vi "AnVOR.vi"() -> ()   [LabVIEW 2013]
uses:
  <vilib>/vision/Measure.llb/Straight Edge Options.ctl
  <vilib>/vision/Measure.llb/Straight Edge Process.ctl
  <vilib>/vision/Measure.llb/Edge Options.ctl
  <vilib>/vision/Measure.llb/Edge Polarity.ctl
  <vilib>/Utility/error.llb/DialogType.ctl
  <vilib>/Analysis/baseanly.llb/Mean (DBL).vi
  <vilib>/Utility/file.llb/Read From Spreadsheet File (string).vi
  <vilib>/Utility/file.llb/Read From Spreadsheet File (DBL).vi
  <vilib>/Utility/file.llb/Write To Spreadsheet File (string).vi
  <vilib>/Utility/file.llb/Write To Spreadsheet File (DBL).vi
  <vilib>/Waveform/WDTFileIO.llb/ Write Waveforms to File (1D).vi
  <vilib>/vision/NI_Vision_Development_Module.lvlib
  <vilib>/Analysis/NI_AALBase.lvlib
panel:
  out "RawTemp":waveform(dbl)[][](array[waveform])
  out "FittingParameter":T1
  out "Vertical 2":i32
  out "Horizontal 2":i32
  in  "buf_vel_graph":dbl[][](array[numeric])
  in  "Close":bool
  in  "InitialCenter":cluster{dbl, dbl}
  in  "BlobPos_Mrk":cluster{dbl, dbl}[](array[cluster])
  in  "GlobalRect_Matches":sgl[](array[numeric])
  in  "Tab Control":T2(tab)
  in  "Image Flip":u32(ring)=3 items=["Horizontal Flip", "Vertical Flip", "Central Flip", "No Flip"]
  in  "Fit Options (Find Straight Edge 3)":T3={"Number of Lines"=1, "Type"=enum."First Edge Rake", "Min. Score"=1.0, "Max. Score"=1000.0, "Orientation"=0.0, "Angle Range"=60.0, "Angle Tolerance"=1.0, "Step Size"=1, "Min. SNR (db)"=200.0, "Min. Points (%)"=25.0, "Hough Iterations"=5} {"Min. Points (%)" min=0.0 max=100.0; "Min. SNR (db)" min=0.0; "Max. Score" min=0.0 max=1024.0; "Min. Score" min=0.0 max=1024.0 step=1.0}
  in  "Fit Options (Find Straight Edge 2)":T3={"Number of Lines"=1, "Type"=enum."First Edge Rake", "Min. Score"=1.0, "Max. Score"=1000.0, "Orientation"=0.0, "Angle Range"=60.0, "Angle Tolerance"=1.0, "Step Size"=1, "Min. SNR (db)"=200.0, "Min. Points (%)"=25.0, "Hough Iterations"=5} {"Min. Points (%)" min=0.0 max=100.0; "Min. SNR (db)" min=0.0; "Max. Score" min=0.0 max=1024.0; "Min. Score" min=0.0 max=1024.0 step=1.0}
  in  "Marker Edge 3":T7={"Search Direction"=0, "Edge Options"={"Edge Polarity"=0, "Kernel Size"=3, "Width"=1, "Minimum Edge Strength"=100.0, "Interpolation Type"=enum."Zero Order", "Data Processing Method"=enum."Average"}, "Show Search Area"=TRUE, "Show Search Lines"=FALSE, "Show Edges Found"=FALSE, "Show Result"=TRUE, "Search Area Color"=65280, "Search Lines Color"=255, "Edge Locations Color"=16776960, "Result Color"=31231, "Overlay Group Name"=""} {"Search Direction" items=["Left to Right", "Right to Left", "Top to Bottom", "Bottom to Top"]; "Edge Options"."Edge Polarity" items=["All Edges", "Rising Edges", "Falling Edges"]; "Edge Options"."Minimum Edge Strength" format="%.2f"; "Edge Options"."Width" step=2; "Edge Options"."Kernel Size" step=2}
  in  "Marker Edge 2":T7={"Search Direction"=3, "Edge Options"={"Edge Polarity"=0, "Kernel Size"=3, "Width"=1, "Minimum Edge Strength"=100.0, "Interpolation Type"=enum."Zero Order", "Data Processing Method"=enum."Average"}, "Show Search Area"=TRUE, "Show Search Lines"=FALSE, "Show Edges Found"=FALSE, "Show Result"=TRUE, "Search Area Color"=65280, "Search Lines Color"=255, "Edge Locations Color"=16776960, "Result Color"=16774656, "Overlay Group Name"=""} {"Search Direction" items=["Left to Right", "Right to Left", "Top to Bottom", "Bottom to Top"]; "Edge Options"."Edge Polarity" items=["All Edges", "Rising Edges", "Falling Edges"]; "Edge Options"."Minimum Edge Strength" format="%.2f"; "Edge Options"."Width" step=2; "Edge Options"."Kernel Size" step=2}
  out "Freq:":string
  in  "FPS:":u32
  in  "CalVar_VA":path caption="Calibration File:"
  in  "Y-axis":dbl=6.0
  in  "X-axis":dbl=6.0
  in  "Cal_Val:":u16(ring) items=["2013-07-05", "2012-08-30", "2012-08-30", "2012-03-17", "2012-03-16", "2012-03-15"]
  out "comp_XY":cluster{"mean":dbl, "mean":dbl, "Angle":sgl}(graph)
  in  "BCGTD":T8={"Brightness"=171.0, "Contrast"=89.0, "Gamma"=2.0, "Detection Sensitivity"=302.0} {"Detection Sensitivity" min=0 max=500 step=1 scale=0.0..500.0 scale format="%.2f"; "Gamma" min=0.1 max=10 step=0.01 scale=0.1..10.0 scale format="%.1f"; "Contrast" min=1 max=89 step=0.1 scale=0.0..89.0 scale format="%.2f"; "Brightness" min=0 max=255 step=1 scale=0.0..255.0 scale format="%.2f"}
  in  "btn_Pause":bool
  in  "btn_SaveResult":bool
  in  "btn_Reset":bool
  in  "btn_Start":bool
  in  "btn_Stop":bool
  in  "btn_Detect":bool
  in  "FrameNum":u32(slide) max=10490 scale=0.0..10490.0
  out "Img_Marker":T9(plugin-control)
  out "Img_Mod":T9(plugin-control)
  out "Img_Org":T9(plugin-control)
  in  "Video File":path
  out "Number of Matches (Pattern Matching 1)":bool
  in  "Fit Options (Find Straight Edge 1)":T3={"Number of Lines"=1, "Type"=enum."First Edge Rake", "Min. Score"=1.0, "Max. Score"=1000.0, "Orientation"=0.0, "Angle Range"=60.0, "Angle Tolerance"=1.0, "Step Size"=1, "Min. SNR (db)"=200.0, "Min. Points (%)"=25.0, "Hough Iterations"=5} {"Min. Points (%)" min=0.0 max=100.0; "Min. SNR (db)" min=0.0; "Max. Score" min=0.0 max=1024.0; "Min. Score" min=0.0 max=1024.0 step=1.0}
  in  "Marker Edge 1":T7={"Search Direction"=2, "Edge Options"={"Edge Polarity"=0, "Kernel Size"=3, "Width"=1, "Minimum Edge Strength"=100.0, "Interpolation Type"=enum."Zero Order", "Data Processing Method"=enum."Average"}, "Show Search Area"=TRUE, "Show Search Lines"=FALSE, "Show Edges Found"=FALSE, "Show Result"=TRUE, "Search Area Color"=65280, "Search Lines Color"=255, "Edge Locations Color"=16776960, "Result Color"=16711680, "Overlay Group Name"=""} {"Search Direction" items=["Left to Right", "Right to Left", "Top to Bottom", "Bottom to Top"]; "Edge Options"."Edge Polarity" items=["All Edges", "Rising Edges", "Falling Edges"]; "Edge Options"."Minimum Edge Strength" format="%.2f"; "Edge Options"."Width" step=2; "Edge Options"."Kernel Size" step=2}
  in  "Round Marker?":bool
  in  "btn_Undo":bool
  in  "Ring":u16(ring)=5 items=["HOR"=5, "VER"=6, "TOR"=7]
  in  "Point Removal":bool
  in  "Averaging Filter":enum32{"Hor", "Ver", "Tor"}(tab)
  in  "HorPk Width":i32(slide)=2 scale=0.0..30.0
  in  "HorL_Threshold":dbl
  in  "HorR_Threshold":dbl
  in  "VerL_Threshold":dbl
  in  "VerR_Threshold":dbl
  in  "VerPk Width":i32(slide)=2 scale=0.0..30.0
  in  "TorL_Threshold":dbl
  in  "TorR_Threshold":dbl
  in  "TorPk Width 3":i32(slide)=2 scale=0.0..30.0
  in  "Img_Only":bool
  in  "Tab Control 3":enum32{"Raw", "Hor_Vel", "Ver_Vel", "Tor_Vel"}(tab)
  out "Grp_ExtPos":waveform(dbl)[](graph)
  out "Grp_ExtVel":waveform(dbl)[](graph)
  in  "filterRank 2":i32=15 min=1
  out "Decaytime (Sec)":dbl
  out "Grp_ExtVel_Hor":waveform(dbl)[](graph)
  out "Grp_CycleAnal_Hor":waveform(dbl)[](graph)
  in  "Enum":enum16{"fromZero", "fromMaximum"}(ring)
  in  "filterRank":i32=20 min=1
  in  "Filp":bool
  out "Grp_ExtVel_Ver":waveform(dbl)[](graph)
  out "Grp_CycleAnal_Ver":waveform(dbl)[](graph)
  out "Grp_ExtVel_Tor":waveform(dbl)[](graph)
  out "Grp_CycleAnal_Tor":waveform(dbl)[](graph)
  in  "Tab Control 2":T10(tab)
  out "AMHV":dbl caption="MHV" format="%0.2f"
  out "#Cycles":dbl
  out "period":dbl caption="Freq" format="%.2g"
  out "Table":string[][](table)
  out "Table 2":string[][](table)
  in  "btn_Analyze":bool
  out "grph_RawPos":dbl[][](graph)
  in  "btn_Remove":bool
  in  "Raw Location:":path
  in  "Raw Data:":i32(listbox)
  in  "X-axis 2":dbl=6.0 caption="X:"
  in  "Y-axis 2":dbl=6.0 caption="Y:"
  in  "CalVar_GA":path caption="Calibration File:"
  in  "Cal_Val: 2":u16(ring) items=["2013-07-05", "2012-08-30", "2012-08-30", "2012-03-17", "2012-03-16", "2012-03-15"]
  in  "btn_SaveAnResult":bool
  in  "Filter Intensity":enum16{"0", "1", "2", "3", "4", "5"}(ring)
  out "Grp_Raw":waveform(dbl)[](graph)
  in  "Analyzed Data:":i32(listbox)
  in  "Final Location: 2":path
  out "x > 0?":bool
  in  "Cutoff?":bool
  in  "# of terms":i32=1
  out "Frequencies":dbl[](array[numeric]) format="%.2f"
  in  "index":i32=3 min=1 max=8
  in  "테이블 컨트롤":string[][](table)
  in  "Axis":u16(ring) items=["Horizontal", "Vertical"]
  in  "btn_addAvg":bool
  in  "Calibration Data:":i32(listbox)
  in  "Calibration Data Location":path
  out "grph_Calibration":waveform(dbl)(graph)
  in  "btn_rmvAvg":bool
  in  "btn_Calculate":bool
  in  "Horizontal":dbl
  in  "Vertical":dbl
  in  "CalVar_Cal":path caption="Calibration File:"
  out "CalList":i32(listbox)
  in  "btn_add2list":bool
  in  "btn_up":bool
  in  "btn_dn":bool
  in  "btn_del":bool
  in  "btn_save":bool
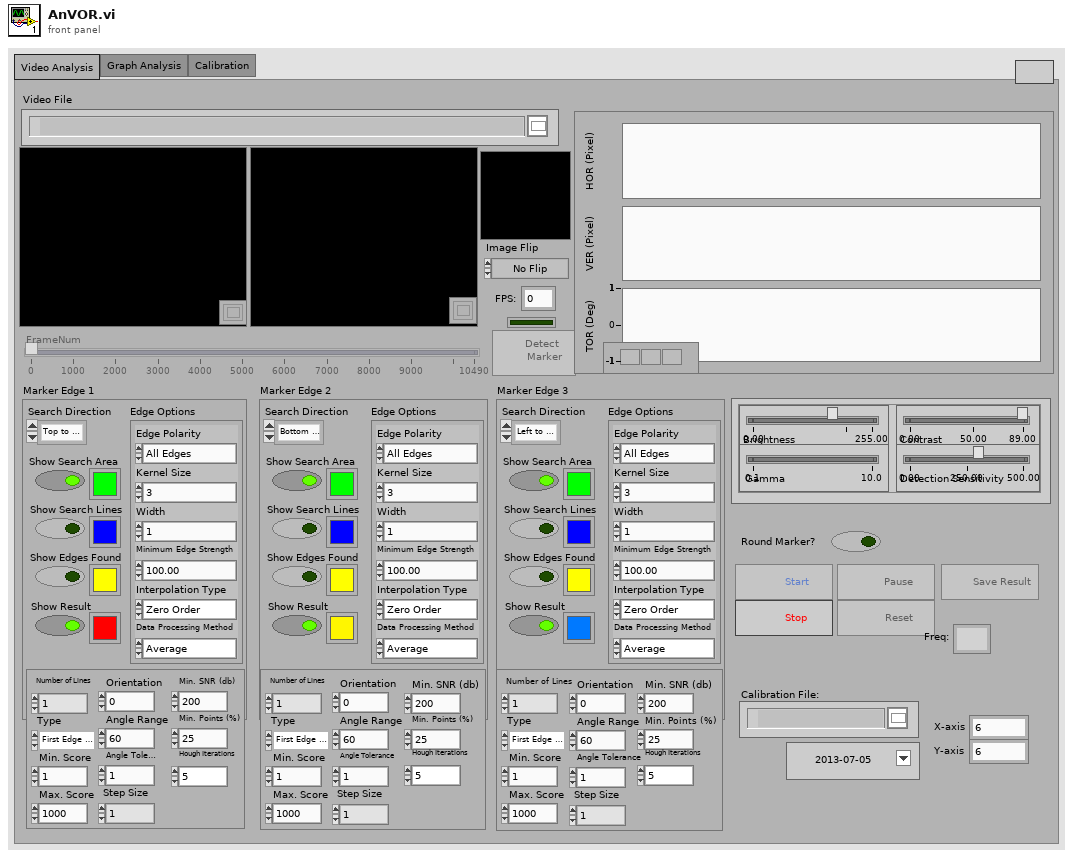
[diagram p1: front panel]
types:
  T1 = cluster{"HorL_Threshold":dbl, "HorR_Threshold":dbl, "HorPk Width":i32, "VerL_Threshold":dbl, "VerR_Threshold":dbl, "VerPk Width":i32, "TorL_Threshold 3":dbl, "TorR_Threshold":dbl, "TorPk Width 3":i32}
  T2 = enum32{"Video Analysis", "Graph Analysis", "Calibration"}
  T3 = typedef "Straight Edge Options.ctl" = cluster{"Number of Lines":i32, "Type":T4, "Min. Score":dbl, "Max. Score":dbl, "Orientation":dbl, "Angle Range":dbl, "Angle Tolerance":dbl, "Step Size":u32, "Min. SNR (db)":dbl, "Min. Points (%)":dbl, "Hough Iterations":i32}
  T4 = typedef "Straight Edge Process.ctl" = enum32{"First Edge Rake", "Best Edge Rake", "Hough Edge Rake", "First Edge Projection", "Best Edge Projection"}
  T5 = typedef "Edge Options.ctl" = cluster{"Edge Polarity":T6, "Kernel Size":u32, "Width":u32, "Minimum Edge Strength":sgl, "Interpolation Type":enum32{"Zero Order", "Bilinear", "Quadratic", "Cubic", "Bilinear Fixed"}, "Data Processing Method":enum32{"Average", "Median"}}
  T6 = typedef "Edge Polarity.ctl" = u32
  T7 = cluster{"Search Direction":u32, "Edge Options":T5, "Show Search Area":bool, "Show Search Lines":bool, "Show Edges Found":bool, "Show Result":bool, "Search Area Color":u32, "Search Lines Color":u32, "Edge Locations Color":u32, "Result Color":u32, "Overlay Group Name":string}
  T8 = cluster{"Brightness":sgl, "Contrast":sgl, "Gamma":sgl, "Detection Sensitivity":sgl}
  T9 = typedef "IMAQ Image.ctl" = refnum<image>
  T10 = enum32{"3D Analysis", "Spontaneous Nystagmus Analysis"}
  T11 = enum16{"RawDataOpen", "FinalDataOpen", "Cal2DateChange", "Calvar2Open", "RawGrpOpen", "FinalGrpOpen", "SelGrp", "RmvGrp", "SaveAnResult", "DetectMarker", "SelPlot", "Undo"}
  T12 = enum16{"Calvar3Open", "CalDataOpen", "CalGrpOpen", "AddAvg", "RmvAvg", "CalCalvar", "AddVar", "SaveVar", "Up", "Dn", "Del"}
  T13 = enum16{"VideoFileOpen", "CalvarOpen", "CalDateChange", "Adj_BCGTD", "StartTrack", "SaveResult"}
  T14 = cluster{"New Image":T9, "New Image":T9, "New Image":T9, "New Image":T9, "New Image":T9}
  T15 = typedef "LVRowAndColumnTypeDef.ctl" = cluster{"Row":i32, "Column":i32}
  T16 = typedef "DialogType.ctl" = u16
  T17 = enum16{"RawDataOpen", "FinalDataOpen", "Cal2DateChange", "Calvar2Open", "RawGrpOpen", "FinalGrpOpen", "SelGrp", "RmvGrp", "SaveAnResult", "DetectMarker", "SelPlot"}
  T18 = cluster{"Global Rectangle":i32[], "Contours":cluster{"Contour Type":u32, "ROI Type":u32, "Points":i32[]}[]}
  T19 = enum8{"Enabled", "Disabled", "Disabled and Grayed Out"}
  T20 = typedef "LVCursorListTypeDef.ctl" = cluster{"Name":string, "Color":u32, "Style":u8, "Point Style":u8, "Name Visible":bool, "Allow Drag":bool, "Cursor Mode":u32, "Plot":i32, "Index":i32, "Position":cluster{"X":dbl, "Y":dbl}, "X Scale":u32, "Y Scale":u32, "Watch Plots":i32[], "Watch All Plots":bool, "Plot Area":i32, "Label Offset":cluster{"X":dbl, "Y":dbl}}[]
  T21 = cluster{"Name":string, "Color":u32, "Style":u8, "Point Style":u8, "Name Visible":bool, "Allow Drag":bool, "Cursor Mode":u32, "Plot":i32, "Index":i32, "Position":cluster{"X":dbl, "Y":dbl}, "X Scale":u32, "Y Scale":u32, "Watch Plots":i32[], "Watch All Plots":bool, "Plot Area":i32, "Label Offset":cluster{"X":dbl, "Y":dbl}}
  T22 = cluster{"Name":string, "Color":u32, "Style":u8, "Point Style":u8, "Name Visible":bool, "Allow Drag":bool, "Cursor Mode":u32, "Plot":i32, "Index":i32, cluster{dbl, "Y":dbl}, "X Scale":u32, "Y Scale":u32, "Watch Plots":i32[], "Watch All Plots":bool, "Plot Area":i32, "Label Offset":cluster{"X":dbl, "Y":dbl}}
  T23 = cluster{"Name":string, "Color":u32, "Style":u8, "Point Style":u8, "Name Visible":bool, "Allow Drag":bool, "Cursor Mode":u32, "Plot":i32, "Index":i32, cluster{dbl, "Y":dbl}, "X Scale":u32, "Y Scale":u32, "Watch Plots":i32[], "Watch All Plots":bool, "Plot Area":i32, "Label Offset":cluster{"X":dbl, "Y":dbl}}[]
  T24 = cluster{dbl, dbl, dbl, dbl, dbl, dbl, dbl, dbl, dbl}
  T25 = enum16{"RawDataOpen", "FinalDataOpen", "Cal2DateChange", "Calvar2Open", "RawGrpOpen", "FinalGrpOpen", "SelGrp", "RmvGrp", "SaveAnResult", "DetectMarker"}
  T26 = typedef "IMAQ Rectangle" = cluster{"Left":i32, "Top":i32, "Right":i32, "Bottom":i32, "Rotation":dbl}
  T27 = typedef "AviRefnum.ctl" = refnum<k1>
  T28 = cluster{"width":u32, "height":u32, "framesPerSecond":u32, "compressionFilter":string, "hasData":bool}
  T29 = cluster{"Brightness":sgl, "Contrast":sgl, "Gamma":sgl}
  T30 = cluster{"Position":cluster{"x":sgl, "y":sgl}, "Angle":sgl, "Scale":sgl, "Score":sgl, "Bounding Box":cluster{"x":sgl, "y":sgl}[]}[]
  T31 = cluster{"Position":cluster{"x":sgl, "y":sgl}, "Angle":sgl, "Scale":sgl, "Score":sgl, "Bounding Box":cluster{"x":sgl, "y":sgl}[]}
  T32 = typedef "ROI Descriptor" = cluster{"Global Rectangle":i32[], "Contours":cluster{"ID":enum32{"External", "Internal"}, "Type":u32, "Coordinates":i32[]}[]}
  T33 = cluster{"Point1 (Pixels)":cluster{"X":sgl, "Y":sgl}, "Point2 (Pixels)":cluster{"X":sgl, "Y":sgl}, "Point1 (Real-World)":cluster{"X":sgl, "Y":sgl}, "Point2 (Real-World)":cluster{"X":sgl, "Y":sgl}, "Angle (Pixel)":dbl, "Angle (Real-World)":dbl, "Score":dbl, "Straightness":dbl, "Average SNR (db)":dbl, "Calibration Valid":bool}
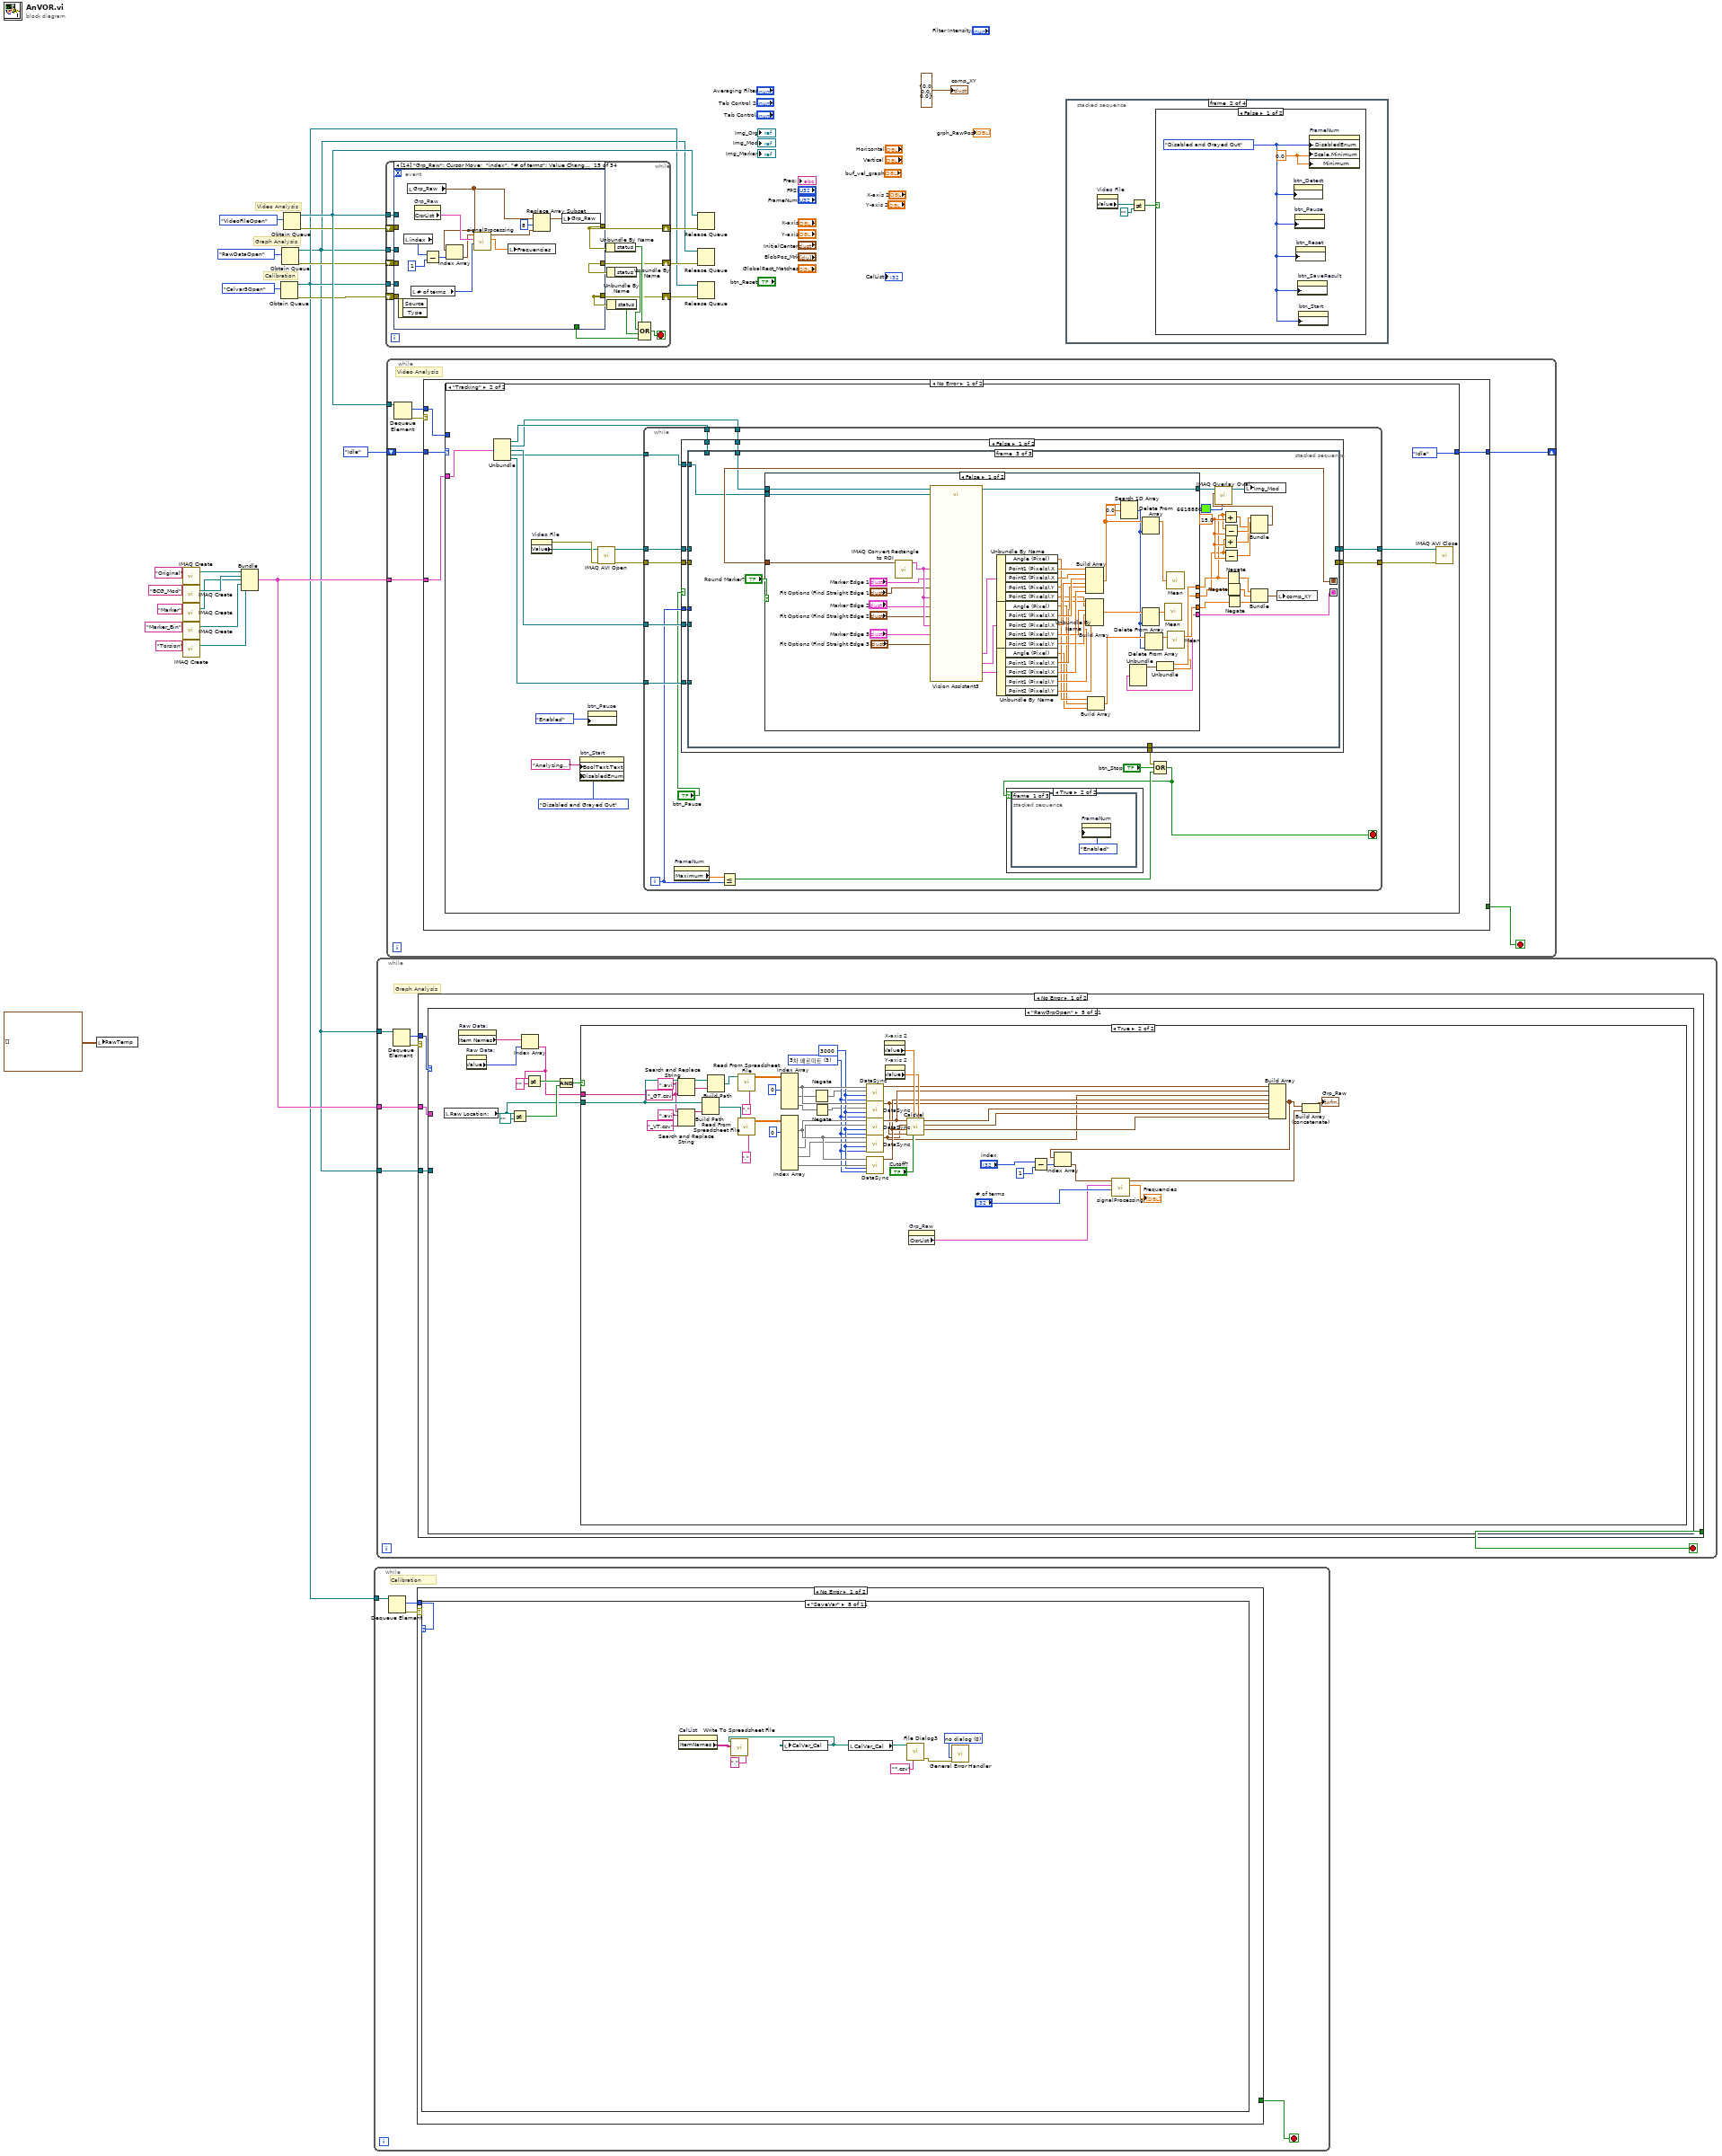
[diagram p0: block diagram]
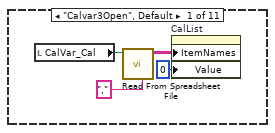
[diagram p2: hidden frame]
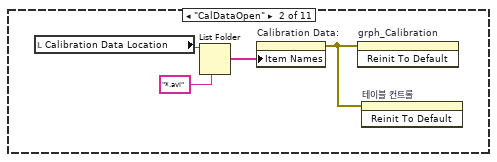
[diagram p3: hidden frame]
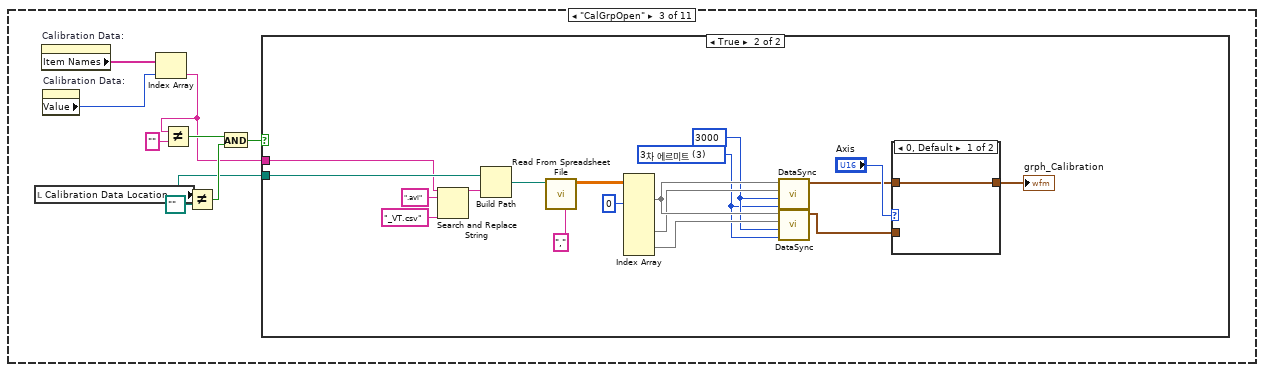
[diagram p4: hidden frame]
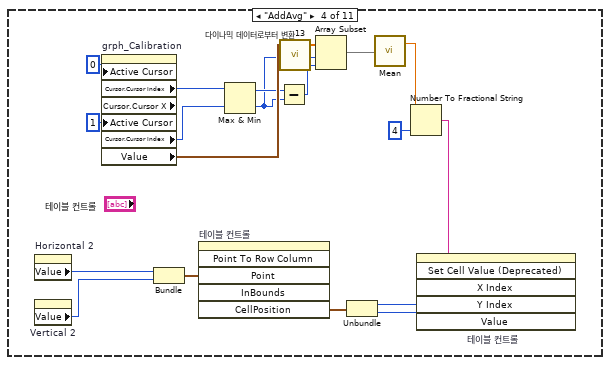
[diagram p7: hidden frame]
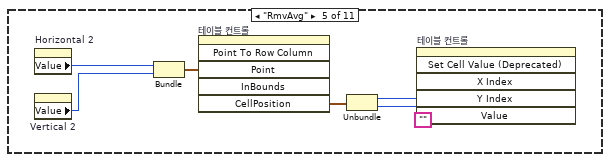
[diagram p8: hidden frame]
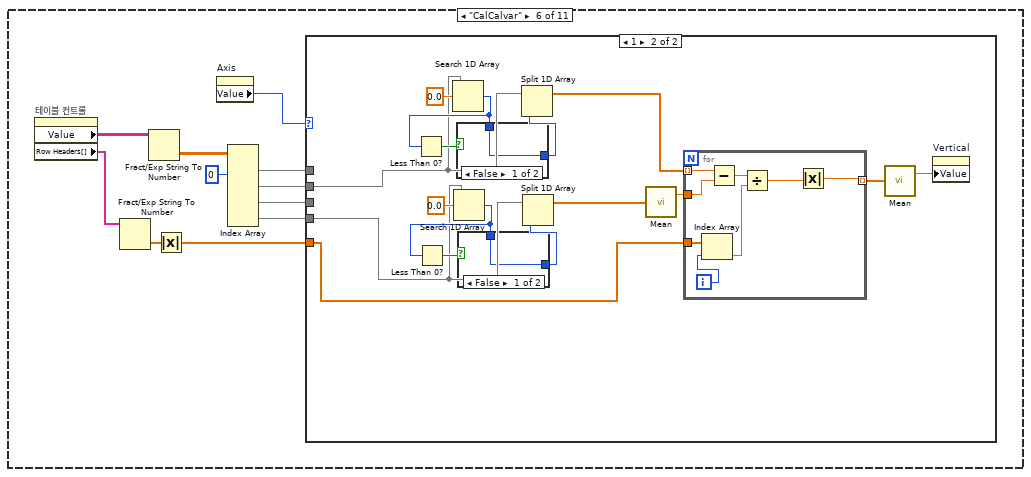
[diagram p9: hidden frame]
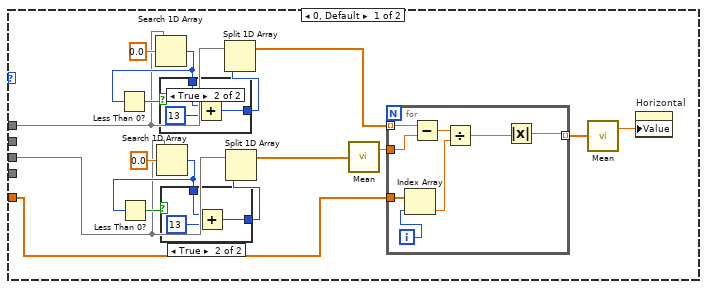
[diagram p10: hidden frame]
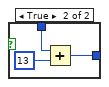
[diagram p13: hidden frame]
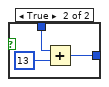
[diagram p14: hidden frame]
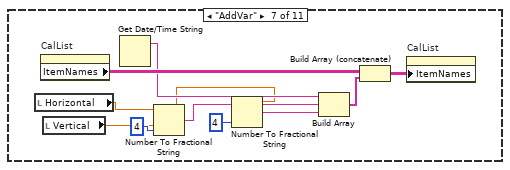
[diagram p15: hidden frame]
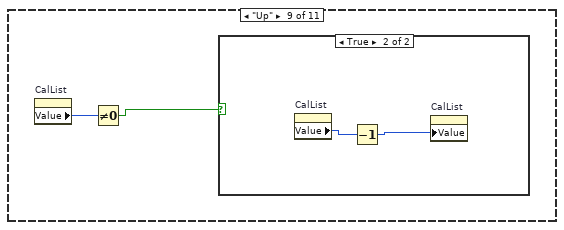
[diagram p16: hidden frame]
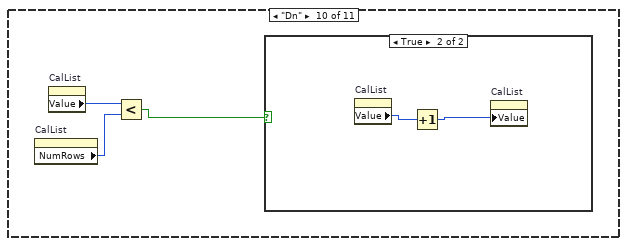
[diagram p18: hidden frame]
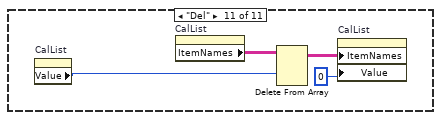
[diagram p20: hidden frame]
diagram:
  # "Calibration"
  # "Graph Analysis"
  # "Video Analysis"
  n1 = local write "RawTemp"(waveform(dbl)[][] [] ("RawTemp")) -> ()
  n2 = call "IMAQ Create"("Image Name"="Original") -> ("New Image"=w12:T9)  [unwired: 3 in, 2 out]
  n3 = call "IMAQ Create"("Image Name"="BCG_Mod") -> ("New Image"=w11:T9)  [unwired: 3 in, 2 out]
  n4 = call "IMAQ Create"("Image Name"="Marker") -> ("New Image"=w10:T9)  [unwired: 3 in, 2 out]
  n5 = call "IMAQ Create"("Image Name"="Marker_Bin") -> ("New Image"=w9:T9)  [unwired: 3 in, 2 out]
  n6 = call "IMAQ Create"("Image Name"="Torsion") -> ("New Image"=w8:T9)  [unwired: 3 in, 2 out]
  n7 = Bundle("New Image"=w12, "New Image"=w11, "New Image"=w10, "New Image"=w9, "New Image"=w8) -> (w7:T14)  [unwired: 1 in]
  n8 = Obtain Queue(element data type=T12."Calvar3Open" ("Enum")) -> (queue out=w4:refnum<queue>, error out=w16:errorcluster)  [unwired: 4 in, 1 out]
  n9 = Obtain Queue(element data type=T11."RawDataOpen" ("Enum")) -> (queue out=w3:refnum<queue>, error out=w17:errorcluster)  [unwired: 4 in, 1 out]
  n10 = Obtain Queue(element data type=T13."VideoFileOpen" ("Enum")) -> (queue out=w21:refnum<queue>, error out=w19:errorcluster)  [unwired: 4 in, 1 out]
  n11 = while {
    tunnel: w4 -> [w30]
    stop <- w27 stop-if-true
    # "Calibration"
    n12 = Dequeue Element(queue=w30) -> (element=w28:T12, error out=w29:errorcluster)  [unwired: 2 in, 2 out]
    n13 = case shown="No Error" w29 {
      tunnel: w28 -> [w31 _]
      tunnel: [_ TRUE] -> w27
      frame No Error {
        n14 = case shown="\"SaveVar\"" w31 {
          frame "Calvar3Open", Default {
            n15 = local read "CalVar_Cal"() -> (w32:path)
            n16 = call-poly <vilib>:"Read From Spreadsheet File.vi"("delimiter (\\t)"="," ("delimiter (\\t)"), "file path (dialog if empty)"=w32) -> ("all rows"=w34:string[][])  [unwired: 5 in, 4 out]
            n17 = property on="CalList" class="MCListbox (strict)"("ItemNames"=w34, "Value"=0 ("CalList")) -> ()  [unwired: 2 in, 2 out]
          }
          frame "CalDataOpen" {
            n18 = local read "Calibration Data Location"() -> (w39:path)
            n19 = List Folder(path=w39, pattern="*.avi") -> (filenames=w38:string[])  [unwired: 2 in, 3 out]
            n20 = property on="Calibration Data:" class="LstBox (strict)"("Item Names"=w38) -> (error out=w36:errorcluster)  [unwired: 2 in, 1 out]
            n21 = invoke on="grph_Calibration" class="WFGraph (엄격한)" method="Reinit To Default"(error in=w36) -> ()  [unwired: 2 in, 3 out]
            n22 = invoke on="테이블 컨트롤" class="Tbl (엄격한)" method="Reinit To Default"(error in=w36) -> ()  [unwired: 2 in, 3 out]
          }
          frame "CalGrpOpen" {
            n23 = local read "Calibration Data Location"() -> (w41:path)
            n24 = property on="Calibration Data:" class="LstBox (strict)"() -> ("Item Names"=w48:string[])  [unwired: 2 in, 2 out]
            n25 = property on="Calibration Data:" class="LstBox (strict)"() -> ("Value"=w42:i32)  [unwired: 2 in, 2 out]
            n26 = Index Array(array=w48, index=w42) -> (element=w40:string)
            n27 = Not Equal?(x=w40, y="") -> (x != y?=w45:bool)
            n28 = Not Equal?(x=w41, y=path "") -> (x != y?=w44:bool)
            n29 = And(x=w45, y=w44) -> (x .and. y?=w43:bool)
            n30 = case shown="True" w43 {
              tunnel: w41 -> [_ w66]
              tunnel: w40 -> [_ w65]
              frame False {
              }
              frame True {
                w53 = 3 items=["최근접", "선형", "스플라인", "3차 에르미트", "라그랑지"] ("method")
                w54 = 3000 ("samples")
                n31 = Search and Replace String(input string=w65, search string=".avi", replace string="_VT.csv" ("replace string (\"\")")) -> (result string=w64:string)  [unwired: 5 in, 3 out]
                n32 = Build Path(base path=w66, name or relative path=w64) -> (appended path=w60:path)
                n33 = call-poly <vilib>:"Read From Spreadsheet File.vi"("delimiter (\\t)"="," ("delimiter (\\t)"), "file path (dialog if empty)"=w60) -> ("all rows"=w59:dbl[][])  [unwired: 5 in, 4 out]
                n34 = Index Array(array=w59, index (col) #1=0 ("disabled index (col)")) -> (element #1=w57:dbl[], element #3=w56:dbl[], element #4=w55:dbl[])  [unwired: 7 in, 1 out]
                n35 = call "DataSync.vi"("method"=w53, "samples"=w54, "Y"=w56, "X"=w57) -> ("출력 웨이브폼"=w51:waveform(dbl))  [unwired: 5 in, 2 out]
                n36 = call "DataSync.vi"("method"=w53, "samples"=w54, "Y"=w55, "X"=w57) -> ("출력 웨이브폼"=w49:waveform(dbl))  [unwired: 5 in, 2 out]
                n37 = case shown="0, Default" "Axis" {
                  tunnel: [w67 w68] -> w50
                  tunnel: w51 -> [w67 _]
                  tunnel: w49 -> [_ w68]
                  frame 0, Default {
                  }
                  frame 1 {
                  }
                }
                "grph_Calibration" <- w50
              }
            }
          }
          frame "AddAvg" {
            n38 = property on="Horizontal 2" class="DigNum (strict)"() -> ("Value"=w73:i32)  [unwired: 2 in, 2 out]
            n39 = property on="Vertical 2" class="DigNum (strict)"() -> ("Value"=w72:i32)  [unwired: 2 in, 2 out]
            n40 = property on="grph_Calibration" class="WFGraph (strict)" props=["Active Cursor", "Cursor", "Cursor Index", "Cursor", "Cursor X", "Active Cursor", "Cursor", "Cursor Index", "Value"]("Active Cursor"=u32 0, "Active Cursor"=u32 1) -> ("Cursor.Cursor Index"=w83:i32, "Cursor.Cursor Index"=w85:i32, "Value"=w84:waveform(dbl))  [unwired: 2 in, 3 out]
            n41 = Bundle("Value"=w73, "Value"=w72) -> (w74:cluster{"Value":i32, "Value":i32})  [unwired: 1 in]
            n42 = invoke on="테이블 컨트롤" class="Tbl (엄격한)" method="Point To Row Column"("Point"=w74) -> ("CellPosition"=w71:T15)  [unwired: 5 in, 5 out]
            n43 = Max & Min(x=w83, y=w85) -> (max(x,y)=w82:i32, min(x,y)=w76:i32)
            n44 = Subtract(x=w82, y=w76) -> (x-y=w81:i32)
            n45 = call "다이나믹 데이터로부터 변환13"("Dynamic Data Type"=w84) -> ("Array"=w77:dbl[])  [unwired: 3 in]
            n46 = Array Subset(array=w77, index=w76, length=w81) -> (w80:dbl[])
            n47 = Unbundle(w71) -> ("Row"=w70:i32, "Column"=w69:i32)
            n48 = call-poly <vilib>:"Mean.vi"("X"=w80) -> ("mean"=w79:dbl)  [unwired: 1 out]
            n49 = Number To Fractional String(number=w79, precision (6)=i16 4) -> (F-format string=w75:string)  [unwired: 2 in]
            n50 = invoke on="테이블 컨트롤" class="Tbl (엄격한)" method="Set Cell Value (Deprecated)"("X Index"=w69, "Y Index"=w70, "Value"=w75) -> ()  [unwired: 3 in, 6 out]
          }
          frame "RmvAvg" {
            n51 = property on="Horizontal 2" class="DigNum (strict)"() -> ("Value"=w93:i32)  [unwired: 2 in, 2 out]
            n52 = property on="Vertical 2" class="DigNum (strict)"() -> ("Value"=w92:i32)  [unwired: 2 in, 2 out]
            n53 = Bundle("Value"=w93, "Value"=w92) -> (w94:cluster{"Value":i32, "Value":i32})  [unwired: 1 in]
            n54 = invoke on="테이블 컨트롤" class="Tbl (엄격한)" method="Point To Row Column"("Point"=w94) -> ("CellPosition"=w91:T15)  [unwired: 5 in, 5 out]
            n55 = Unbundle(w91) -> ("Row"=w90:i32, "Column"=w89:i32)
            n56 = invoke on="테이블 컨트롤" class="Tbl (엄격한)" method="Set Cell Value (Deprecated)"("X Index"=w89, "Y Index"=w90, "Value"="") -> ()  [unwired: 3 in, 6 out]
          }
          frame "CalCalvar" {
            n57 = property on="테이블 컨트롤" class="Tbl (strict)"() -> ("Value"=w103:string[][], "Row Headers[]"=w101:string[])  [unwired: 2 in, 2 out]
            n58 = Fract/Exp String To Number(string=w101) -> (number=w98:dbl[])  [unwired: 3 in, 1 out]
            n59 = Fract/Exp String To Number(string=w103) -> (number=w102:dbl[][])  [unwired: 3 in, 1 out]
            n60 = Absolute Value(x=w98) -> (abs(x)=w97:dbl[])
            n61 = property on="Axis" class="Ring (strict)"() -> ("Value"=w100:u16)  [unwired: 2 in, 2 out]
            n62 = Index Array(array=w102, index (col) #1=0 ("비활성화된 인덱스 (열)")) -> (element #1=w104:dbl[], element #2=w96:dbl[], element #3=w99:dbl[], element #4=w95:dbl[])  [unwired: 7 in]
            n63 = case shown="1" w100 {
              tunnel: w104 -> [w114 _]
              tunnel: w99 -> [w108 _]
              tunnel: w97 -> [w106 w140]
              tunnel: w96 -> [_ w139]
              tunnel: w95 -> [_ w138]
              frame 0, Default {
                n64 = Search 1D Array(1D array=w114, element=0.0) -> (index of element=w117:i32)  [unwired: 1 in]
                n65 = Less Than 0?(x=w117) -> (x < 0?=w116:bool)
                n66 = Search 1D Array(1D array=w108, element=0.0) -> (index of element=w110:i32)  [unwired: 1 in]
                n67 = Less Than 0?(x=w110) -> (x < 0?=w111:bool)
                n68 = case shown="True" w116 {
                  tunnel: w117 -> [w126 w129]
                  tunnel: [w126 w127] -> w118
                  frame False {
                  }
                  frame True {
                    n69 = Add(x=w129, y=13) -> (x+y=w127:i32)
                  }
                }
                n70 = case shown="True" w111 {
                  tunnel: w110 -> [w122 w125]
                  tunnel: [w122 w123] -> w109
                  frame False {
                  }
                  frame True {
                    n71 = Add(x=w125, y=13) -> (x+y=w123:i32)
                  }
                }
                n72 = Split 1D Array(array=w114, index=w118) -> (first subarray=w113:dbl[])  [unwired: 1 out]
                n73 = Split 1D Array(array=w108, index=w109) -> (first subarray=w107:dbl[])  [unwired: 1 out]
                n74 = call-poly <vilib>:"Mean.vi"("X"=w107) -> ("mean"=w121:dbl)  [unwired: 1 out]
                n75 = for {
                  tunnel: w113 -> [w137] mode=indexing
                  tunnel: w121 -> [w136]
                  tunnel: w106 -> [w134]
                  tunnel: [w130] -> w120 mode=indexing
                  i -> [w133]
                  n76 = Index Array(array=w134, index=w133) -> (element=w132:dbl)
                  n77 = Subtract(x=w137, y=w136) -> (x-y=w135:dbl)
                  n78 = Divide(x=w135, y=w132) -> (x/y=w131:dbl)
                  n79 = Absolute Value(x=w131) -> (abs(x)=w130:dbl)
                }
                n80 = call-poly <vilib>:"Mean.vi"("X"=w120) -> ("mean"=w119:dbl)  [unwired: 1 out]
                n81 = property on="Horizontal" class="DigNum (strict)"("Value"=w119) -> ()  [unwired: 2 in, 2 out]
              }
              frame 1 {
                n82 = Search 1D Array(1D array=w139, element=0.0) -> (index of element=w149:i32)  [unwired: 1 in]
                n83 = Less Than 0?(x=w149) -> (x < 0?=w148:bool)
                n84 = Search 1D Array(1D array=w138, element=0.0) -> (index of element=w143:i32)  [unwired: 1 in]
                n85 = Less Than 0?(x=w143) -> (x < 0?=w144:bool)
                n86 = case shown="False" w148 {
                  tunnel: w149 -> [w158 w161]
                  tunnel: [w158 w159] -> w150
                  frame False {
                  }
                  frame True {
                    n87 = Add(x=w161, y=13) -> (x+y=w159:i32)
                  }
                }
                n88 = case shown="False" w144 {
                  tunnel: w143 -> [w154 w157]
                  tunnel: [w154 w155] -> w142
                  frame False {
                  }
                  frame True {
                    n89 = Add(x=w157, y=13) -> (x+y=w155:i32)
                  }
                }
                n90 = Split 1D Array(array=w139, index=w150) -> (first subarray=w146:dbl[])  [unwired: 1 out]
                n91 = Split 1D Array(array=w138, index=w142) -> (first subarray=w141:dbl[])  [unwired: 1 out]
                n92 = call-poly <vilib>:"Mean.vi"("X"=w141) -> ("mean"=w153:dbl)  [unwired: 1 out]
                n93 = for {
                  tunnel: w146 -> [w169] mode=indexing
                  tunnel: w153 -> [w168]
                  tunnel: w140 -> [w166]
                  tunnel: [w163] -> w152 mode=indexing
                  i -> [w165]
                  n94 = Index Array(array=w166, index=w165) -> (element=w164:dbl)
                  n95 = Subtract(x=w169, y=w168) -> (x-y=w167:dbl)
                  n96 = Divide(x=w167, y=w164) -> (x/y=w162:dbl)
                  n97 = Absolute Value(x=w162) -> (abs(x)=w163:dbl)
                }
                n98 = call-poly <vilib>:"Mean.vi"("X"=w152) -> ("mean"=w151:dbl)  [unwired: 1 out]
                n99 = property on="Vertical" class="DigNum (strict)"("Value"=w151) -> ()  [unwired: 2 in, 2 out]
              }
            }
          }
          frame "AddVar" {
            n100 = local read "Horizontal"() -> (w177:dbl)
            n101 = property on="CalList" class="MCListbox (strict)"() -> ("ItemNames"=w179:string[][])  [unwired: 2 in, 2 out]
            n102 = local read "Vertical"() -> (w174:dbl)
            n103 = Get Date/Time String() -> (date string=w178:string)  [unwired: 3 in, 1 out]
            n104 = Number To Fractional String(number=w177, precision (6)=i16 4) -> (F-format string=w173:string)  [unwired: 2 in]
            n105 = Number To Fractional String(number=w174, precision (6)=i16 4) -> (F-format string=w172:string)  [unwired: 2 in]
            n106 = Build Array(w178, w173, w172) -> (w171:string[])
            n107 = Build Array (concatenate)(w179, w171) -> (w170:string[][])
            n108 = property on="CalList" class="MCListbox (strict)"("ItemNames"=w170) -> ()  [unwired: 2 in, 2 out]
          }
          frame "SaveVar" {
            w181 = T16 0 items=["no dialog", "OK message", "continue or stop message", "OK message + warnings", "continue/stop + warnings"] ("type of dialog (OK msg:1)")
            n109 = property on="CalList" class="MCListbox (strict)"() -> ("ItemNames"=w186:string[][])  [unwired: 2 in, 2 out]
            n110 = local read "CalVar_Cal"() -> (w184:path)
            n111 = call "File Dialog3"("start path"=w184, "pattern (all files)"="*.csv") -> ("selected path"=w180:path, "error out"=w182:errorcluster)  [unwired: 10 in, 2 out]
            n112 = call-poly <vilib>:"Write To Spreadsheet File.vi"("delimiter (\\t)"="," ("delimiter (\\t)"), "2D data"=w186, "file path (dialog if empty)"=w180) -> ()  [unwired: 5 in, 1 out]
            n113 = local write "CalVar_Cal"(w180) -> ()
            n114 = call <vilib>:"General Error Handler.vi"("type of dialog (OK msg:1)"=w181, "error in (no error)"=w182) -> ()  [unwired: 9 in, 5 out]
          }
          frame "Up" {
            n115 = property on="CalList" class="MCListbox (strict)"() -> ("Value"=w188:i32)  [unwired: 2 in, 2 out]
            n116 = Not Equal To 0?(x=w188) -> (x != 0?=w187:bool)
            n117 = case shown="True" w187 {
              frame False {
              }
              frame True {
                n118 = property on="CalList" class="MCListbox (strict)"() -> ("Value"=w190:i32)  [unwired: 2 in, 2 out]
                n119 = Decrement(x=w190) -> (x-1=w189:i32)
                n120 = property on="CalList" class="MCListbox (strict)"("Value"=w189) -> ()  [unwired: 2 in, 2 out]
              }
            }
          }
          frame "Dn" {
            n121 = property on="CalList" class="MCListbox (strict)"() -> ("NumRows"=w192:u32)  [unwired: 2 in, 2 out]
            n122 = property on="CalList" class="MCListbox (strict)"() -> ("Value"=w193:i32)  [unwired: 2 in, 2 out]
            n123 = Less?(x=w193, y=w192) -> (x < y?=w191:bool)
            n124 = case shown="True" w191 {
              frame False {
              }
              frame True {
                n125 = property on="CalList" class="MCListbox (strict)"() -> ("Value"=w195:i32)  [unwired: 2 in, 2 out]
                n126 = Increment(x=w195) -> (x+1=w194:i32)
                n127 = property on="CalList" class="MCListbox (strict)"("Value"=w194) -> ()  [unwired: 2 in, 2 out]
              }
            }
          }
          frame "Del" {
            n128 = property on="CalList" class="MCListbox (strict)"() -> ("Value"=w196:i32)  [unwired: 2 in, 2 out]
            n129 = property on="CalList" class="MCListbox (strict)"() -> ("ItemNames"=w199:string[][])  [unwired: 2 in, 2 out]
            n130 = Delete From Array(array=w199, index (row)=w196) -> (array with subset deleted=w198:string[][])  [unwired: 2 in, 1 out]
            n131 = property on="CalList" class="MCListbox (strict)"("ItemNames"=w198, "Value"=0 ("CalList")) -> ()  [unwired: 2 in, 2 out]
          }
        }
      }
      frame Error {
      }
    }
  }
  n132 = while {
    tunnel: w3 -> [w206]
    tunnel: w7 -> [w202]
    tunnel: w3 -> [w201]
    stop <- w203 stop-if-true
    # "Graph Analysis"
    n133 = Dequeue Element(queue=w206) -> (element=w204:T11, error out=w205:errorcluster)  [unwired: 2 in, 2 out]
    n134 = case shown="No Error" w205 {
      tunnel: w204 -> [w209 _]
      tunnel: [_ TRUE] -> w203
      tunnel: w202 -> [w208 _]
      tunnel: w201 -> [w207 _]
      frame No Error {
        n135 = case shown="\"RawGrpOpen\"" w209 {
          tunnel: w208 -> [_ _ _ _ _ _ w501 _ _ _ _]
          tunnel: w207 -> [_ _ w251 _ _ _ _ w535 _ _ _]
          frame "RawDataOpen", Default {
            n136 = local read "Raw Location:"() -> (w214:path)
            n137 = List Folder(path=w214, pattern="*_GT.csv") -> (filenames=w211:string[])  [unwired: 2 in, 3 out]
            n138 = for {
              tunnel: w211 -> [w216] mode=indexing
              tunnel: [w215] -> w210 mode=indexing
              n139 = Search and Replace String(input string=w216, search string="_GT.csv", replace string=".avi" ("replace string (\"\")")) -> (result string=w215:string)  [unwired: 5 in, 3 out]
            }
            n140 = property on="Raw Data:" class="LstBox (strict)"("Item Names"=w210) -> (error out=w213:errorcluster)  [unwired: 2 in, 1 out]
            n141 = invoke on="buf_vel_graph" class="Arr (strict)" method="Reinit To Default"(error in=w213) -> ()  [unwired: 2 in, 3 out]
          }
          frame "FinalDataOpen" {
            n142 = local read "Final Location: 2"() -> (w219:path)
            n143 = List Folder(path=w219, pattern="*.csv") -> (filenames=w228:string[])  [unwired: 2 in, 3 out]
            n144 = for {
              tunnel: w228 -> [w249] mode=indexing
              tunnel: [w246] -> w222 mode=indexing
              workers-P: _ -> [_]
              n145 = Search and Replace String(input string=w249, search string="_grph") -> (result string=w247:string)  [unwired: 6 in, 3 out]
              n146 = Search and Replace String(input string=w247, search string="_FitPara") -> (result string=w246:string)  [unwired: 6 in, 3 out]
            }
            n147 = Sort 1D Array(array=w222) -> (sorted array=w223:string[])
            n148 = Array Size(array=w222) -> (size(s)=w227:i32)
            n149 = for {
              N: w227 -> [_]
              shift-right: [w234] -> w225
              shift-left: w223 -> [w233]
              shift-right: [w230] -> _
              shift-left: "" -> [w238]
              shift-right: [w235] -> w226
              shift-left: 0 -> [w236]
              i -> [w232]
              stop <- w231 stop-if-true
              n150 = Index Array(array=w233, index=w232) -> (element=w230:string)
              n151 = Not Equal?(x=w230, y=w238) -> (x != y?=w237:bool)
              n152 = case shown="True" w237 {
                tunnel: w236 -> [w240 w244]
                tunnel: [w240 w245] -> w235
                tunnel: w230 -> [_ w243]
                tunnel: w233 -> [w239 w242]
                tunnel: [w239 w241] -> w234
                frame False {
                }
                frame True {
                  n153 = Replace Array Subset(array=w242, new element=w243, index=w244) -> (w241:string[])
                  n154 = Increment(x=w244) -> (x+1=w245:i32)
                }
              }
              n155 = Empty String/Path?(string/path=w230) -> (empty?=w231:bool)
            }
            n156 = Reshape Array(w225, w226) -> (w220:string[])
            n157 = property on="Analyzed Data:" class="LstBox (strict)"("Item Names"=w220) -> ()  [unwired: 2 in, 2 out]
          }
          frame "Cal2DateChange" {
            n158 = local read "CalVar_GA"() -> (w256:path)
            n159 = local read "Cal_Val: 2"() -> (w257:u16)
            n160 = property on="Grp_Raw" class="WFGraph (strict)"() -> ("Value"=w255:waveform(dbl)[])  [unwired: 2 in, 2 out]
            n161 = call "다이나믹 데이터로부터 변환3"("Dynamic Data Type"=w255) -> ("Array"=w254:dbl[])  [unwired: 3 in]
            n162 = Empty Array?(array=w254) -> (empty?=w253:bool)
            n163 = call-poly <vilib>:"Read From Spreadsheet File.vi"("delimiter (\\t)"="," ("delimiter (\\t)"), "file path (dialog if empty)"=w256) -> ("all rows"=w259:dbl[][])  [unwired: 5 in, 4 out]
            n164 = Not(x=w253) -> (.not. x?=w252:bool)
            n165 = case shown="True" w252 {
              tunnel: w251 -> [_ w268]
              frame False {
              }
              frame True {
                n166 = Enqueue Element(queue=w268, element=T17."RawGrpOpen" ("Enum")) -> (error out=w267:errorcluster)  [unwired: 2 in, 2 out]
                n167 = Enqueue Element(queue=w268, element=T17."SelGrp" ("Enum"), error in (no error)=w267) -> ()  [unwired: 1 in, 3 out]
              }
            }
            n168 = Index Array(array=w259, index (col) #1=1 ("disabled index (col)")) -> (element #1=w263:dbl[], element #2=w265:dbl[])  [unwired: 3 in]
            n169 = Reverse 1D Array(array=w263) -> (reversed array=w264:dbl[])
            n170 = Reverse 1D Array(array=w265) -> (reversed array=w266:dbl[])
            n171 = Index Array(array=w264, index=w257) -> (element=w261:dbl)
            n172 = Index Array(array=w266, index=w257) -> (element=w262:dbl)
            n173 = local write "X-axis 2"(w261) -> ()
            n174 = local write "Y-axis 2"(w262) -> ()
          }
          frame "Calvar2Open" {
            n175 = local read "CalVar_GA"() -> (w271:path)
            n176 = call-poly <vilib>:"Read From Spreadsheet File.vi"("delimiter (\\t)"="," ("delimiter (\\t)"), "file path (dialog if empty)"=w271) -> ("all rows"=w279:string[][])  [unwired: 5 in, 4 out]
            n177 = Index Array(array=w279, index (col) #1=0 ("disabled index (col)")) -> (element #1=w277:string[], element #2=w282:string[], element #3=w286:string[])  [unwired: 5 in]
            n178 = Reverse 1D Array(array=w277) -> (reversed array=w281:string[])
            n179 = Reverse 1D Array(array=w282) -> (reversed array=w283:string[])
            n180 = Reverse 1D Array(array=w286) -> (reversed array=w288:string[])
            n181 = Index Array(array=w288, index=0) -> (element=w289:string)
            n182 = Index Array(array=w281, index=0) -> (element=w274:string)
            n183 = Index Array(array=w283, index=0) -> (element=w285:string)
            n184 = property on="Cal_Val: 2" class="Ring (strict)"("Strings []"=w281) -> (error out=w276:errorcluster)  [unwired: 2 in, 1 out]
            n185 = property on="Cal_Val: 2" class="Ring (strict)"(error in=w276, "RingText.Text"=w274) -> ()  [unwired: 1 in, 2 out]
            n186 = Fract/Exp String To Number(string=w285) -> (number=w273:dbl)  [unwired: 3 in, 1 out]
            n187 = Fract/Exp String To Number(string=w289) -> (number=w272:dbl)  [unwired: 3 in, 1 out]
            n188 = local write "Y-axis 2"(w272) -> ()
            n189 = local write "X-axis 2"(w273) -> ()
          }
          frame "RawGrpOpen" {
            n190 = local read "Raw Location:"() -> (w291:path)
            n191 = property on="Raw Data:" class="LstBox (strict)"() -> ("Item Names"=w298:string[])  [unwired: 2 in, 2 out]
            n192 = property on="Raw Data:" class="LstBox (strict)"() -> ("Value"=w292:i32)  [unwired: 2 in, 2 out]
            n193 = Not Equal?(x=w291, y=path "") -> (x != y?=w294:bool)
            n194 = Index Array(array=w298, index=w292) -> (element=w290:string)
            n195 = Not Equal?(x=w290, y="") -> (x != y?=w295:bool)
            n196 = And(x=w295, y=w294) -> (x .and. y?=w293:bool)
            n197 = case shown="True" w293 {
              tunnel: w291 -> [_ w346]
              tunnel: w290 -> [_ w345]
              frame False {
              }
              frame True {
                w322 = 3 items=["최근접", "선형", "스플라인", "3차 에르미트", "라그랑지"] ("method")
                w325 = 3000 ("samples")
                n198 = Search and Replace String(input string=w345, search string=".avi", replace string="_GT.csv" ("replace string (\"\")")) -> (result string=w339:string)  [unwired: 5 in, 3 out]
                n199 = Search and Replace String(input string=w345, search string=".avi", replace string="_VT.csv" ("replace string (\"\")")) -> (result string=w344:string)  [unwired: 5 in, 3 out]
                n200 = Build Path(base path=w346, name or relative path=w344) -> (appended path=w335:path)
                n201 = Build Path(base path=w346, name or relative path=w339) -> (appended path=w337:path)
                n202 = call-poly <vilib>:"Read From Spreadsheet File.vi"("delimiter (\\t)"="," ("delimiter (\\t)"), "file path (dialog if empty)"=w335) -> ("all rows"=w333:dbl[][])  [unwired: 5 in, 4 out]
                n203 = call-poly <vilib>:"Read From Spreadsheet File.vi"("delimiter (\\t)"="," ("delimiter (\\t)"), "file path (dialog if empty)"=w337) -> ("all rows"=w334:dbl[][])  [unwired: 5 in, 4 out]
                n204 = Index Array(array=w334, index (col) #1=0 ("disabled index (col)")) -> (element #1=w330:dbl[], element #2=w320:dbl[], element #3=w319:dbl[])  [unwired: 5 in]
                n205 = Index Array(array=w333, index (col) #1=0 ("disabled index (col)")) -> (element #1=w329:dbl[], element #3=w328:dbl[], element #4=w327:dbl[], element #5=w326:dbl[])  [unwired: 9 in, 1 out]
                n206 = Negate(x=w320) -> (-x=w321:dbl[])
                n207 = Negate(x=w319) -> (-x=w318:dbl[])
                n208 = call "DataSync.vi"("method"=w322, "samples"=w325, "Y"=w321, "X"=w330) -> ("출력 웨이브폼"=w317:waveform(dbl))  [unwired: 5 in, 2 out]
                n209 = call "DataSync.vi"("method"=w322, "samples"=w325, "Y"=w318, "X"=w330) -> ("출력 웨이브폼"=w314:waveform(dbl))  [unwired: 5 in, 2 out]
                n210 = call "DataSync.vi"("method"=w322, "samples"=w325, "Y"=w328, "X"=w329) -> ("출력 웨이브폼"=w316:waveform(dbl))  [unwired: 5 in, 2 out]
                n211 = call "DataSync.vi"("method"=w322, "samples"=w325, "Y"=w327, "X"=w329) -> ("출력 웨이브폼"=w308:waveform(dbl))  [unwired: 5 in, 2 out]
                n212 = call "DataSync.vi"("method"=w322, "samples"=w325, "Y"=w326, "X"=w329) -> ("출력 웨이브폼"=w315:waveform(dbl))  [unwired: 5 in, 2 out]
                n213 = property on="X-axis 2" class="DigNum (strict)"() -> ("Value"=w324:dbl)  [unwired: 2 in, 2 out]
                n214 = property on="Y-axis 2" class="DigNum (strict)"() -> ("Value"=w323:dbl)  [unwired: 2 in, 2 out]
                n215 = call "CalcVel.vi"("CalY"=w323, "Cutoff?"="Cutoff?", "CalX"=w324, "HV"=w314, "Tor"=w315, "Ver"=w308, "Hor"=w316) -> ("TorVel"=w311:waveform(dbl), "VerVel"=w312:waveform(dbl), "HorVel"=w313:waveform(dbl))  [unwired: 2 in]
                n216 = property on="Grp_Raw" class="WFGraph (strict)"() -> ("CrsrList"=w306:T20)  [unwired: 2 in, 2 out]
                n217 = Subtract(x="index", y=1) -> (x-y=w301:i32)
                n218 = Build Array(w317, w316, w308, w315, w314, w313, w312, w311) -> (w303:waveform(dbl)[])
                n219 = Index Array(array=w303, index=w301) -> (element=w302:waveform(dbl))
                n220 = call "signalProcessing.vi"("number of terms"="# of terms", "array"=w306, "waveform in"=w302) -> ("Frequencies"=→"Frequencies":dbl[], "output waveform"=w304:waveform(dbl))  [unwired: 6 in, 1 out]
                n221 = Build Array (concatenate)(w303, w304) -> (→"Grp_Raw":waveform(dbl)[])
              }
            }
          }
          frame "SelGrp" {
            n222 = property on="Filter Intensity" class="Enum (strict)"() -> ("Value"=w470:enum16{"0", "1", "2", "3", "4", "5"})  [unwired: 2 in, 2 out]
            n223 = property on="Grp_Raw" class="WFGraph (strict)"("Active Cursor"=u32 0, "Active Cursor"=u32 1) -> ("Cursor.Cursor X"=w473:dbl, "Cursor.Cursor X"=w472:dbl, "Value"=w471:waveform(dbl)[])  [unwired: 2 in, 2 out]
            n224 = case shown="\"1\"" w470 {
              tunnel: w471 -> [w490 w492 w494 w496 w498 w500]
              tunnel: [w490 w491 w493 w495 w497 w499] -> w469
              frame "0", Default {
              }
              frame "1" {
                n225 = call "필터3"("Signal"=w492) -> ("Filtered Signal"=w491:dynamicdata)  [unwired: 9 in, 1 out]
              }
              frame "2" {
                n226 = call "필터"("Signal"=w494) -> ("Filtered Signal"=w493:dynamicdata)  [unwired: 9 in, 1 out]
              }
              frame "3" {
                n227 = call "필터2"("Signal"=w496) -> ("Filtered Signal"=w495:dynamicdata)  [unwired: 9 in, 1 out]
              }
              frame "4" {
                n228 = call "필터4"("Signal"=w498) -> ("Filtered Signal"=w497:dynamicdata)  [unwired: 9 in, 1 out]
              }
              frame "5" {
                n229 = call "필터5"("Signal"=w500) -> ("Filtered Signal"=w499:dynamicdata)  [unwired: 9 in, 1 out]
              }
            }
            n230 = Max & Min(x=w473, y=w472) -> (max(x,y)=w476:dbl, min(x,y)=w467:dbl)
            n231 = Subtract(x=w476, y=w467) -> (x-y=w468:dbl)
            n232 = Bundle By Name(cluster=T1 {"HorL_Threshold"=0.0, "HorR_Threshold"=0.0, "HorPk Width"=2, "VerL_Threshold"=0.0, "VerR_Threshold"=0.0, "VerPk Width"=2, "TorL_Threshold 3"=0.0, "TorR_Threshold"=0.0, "TorPk Width 3"=2} ("FittingPara"), "HorPk Width"="HorPk Width", "HorR_Threshold"="HorR_Threshold", "HorL_Threshold"="HorL_Threshold", "VerPk Width"="VerPk Width", "VerR_Threshold"="VerR_Threshold", "VerL_Threshold"="VerL_Threshold", "TorPk Width 3"="TorPk Width 3", "TorR_Threshold"="TorR_Threshold", "TorL_Threshold 3"="TorL_Threshold") -> (w439:T1)
            "FittingParameter" <- w439
            n233 = call "AnalyzeGraph.vi"("Grp_Raw"=w469, "start samples/time"=w467, "FittingPara"=w439, "duration"=w468) -> ("Grp_ExtVel"=w459:waveform(dbl)[], "Grp_ExtPos"=→"Grp_ExtPos":waveform(dbl)[], "Hor_CycleOut"=→"Grp_CycleAnal_Hor":waveform(dbl)[], "Table_Out"=w461:dbl[][], "Basic_Detection"=w465:cluster{"period":dbl, "mean":dbl, dbl}, "Ver_CycleOut"=→"Grp_CycleAnal_Ver":waveform(dbl)[], "SNTable_Out"=w450:dbl[][], "Tor_CycleOut"=→"Grp_CycleAnal_Tor":waveform(dbl)[])  [unwired: 2 in, 2 out]
            "Grp_ExtVel" <- w459
            n234 = Unbundle(w465) -> ("period"=→"period":dbl, "mean"=→"AMHV":dbl, →"#Cycles":dbl)
            n235 = Number To Fractional String(number=w461) -> (F-format string=→"Table":string[][])  [unwired: 3 in]
            n236 = Number To Fractional String(number=w450) -> (F-format string=→"Table 2":string[][])  [unwired: 3 in]
            n237 = Index Array(array=w459) -> (element #1=w438:waveform(dbl), element #2=w436:waveform(dbl), element #3=w458:waveform(dbl), element #4=w456:waveform(dbl))  [unwired: 4 in]
            n238 = Build Array(w438, w458) -> (→"Grp_ExtVel_Ver":waveform(dbl)[])
            n239 = Build Array(w438, w456) -> (→"Grp_ExtVel_Tor":waveform(dbl)[])
            n240 = Unbundle By Name(w436) -> ("t0"=w419:timestamp, "dt"=w372:dbl, "Y"=w367:dbl[])
            n241 = Negate(x=w367) -> (-x=w368:dbl[])
            n242 = Select(t=w368, s="Filp", f=w367) -> (s? t:f=w353:dbl[])
            n243 = Index Array(array=w353) -> (element=w418:dbl)  [unwired: 1 in]
            n244 = Array Max & Min(array=w353) -> (max value=w354:dbl)  [unwired: 3 out]
            n245 = for {
              shift-right: [w477] -> _
              shift-left: w418 -> [w479]
              tunnel: w353 -> [w478] mode=indexing
              tunnel: [w477] -> w351 mode=indexing
              n246 = Greater Than 0?(x=w478) -> (x > 0?=w480:bool)
              n247 = Select(t=w479, s=w480, f=w478) -> (s? t:f=w477:dbl)
            }
            n248 = Equal To 0?(x="Enum") -> (x = 0?=w420:bool)
            n249 = Select(t=0.0, s=w420, f=w354) -> (s? t:f=w365:dbl)
            n250 = call "Median.vi"("Rank"="filterRank", "Array in"=w351) -> ("Array out"=w349:dbl[])  [unwired: 9 in]
            n251 = Subtract(x=1.0, y=0.36787944117144233) -> (x-y=w430:dbl)
            n252 = Multiply(x=1.0, y=w349) -> (x*y=w348:dbl[])
            n253 = Negate(x=w365) -> (-x=w366:dbl)
            n254 = Select(t=w366, s="Filp", f=w365) -> (s? t:f=w364:dbl)
            n255 = call "MovingAverage.vi"("Rank"="filterRank 2", "Array in"=w348) -> ("Array out"=w352:dbl[])  [unwired: 9 in]
            n256 = Array Max & Min(array=w352) -> (min value=w361:dbl, min index (indices)=w373:i32)  [unwired: 2 out]
            n257 = Subtract(x=w365, y=w361) -> (x-y=w431:dbl)
            n258 = Multiply(x=w431, y=w430) -> (x*y=w427:dbl)
            n259 = Add(x=w361, y=w427) -> (x+y=w358:dbl)
            n260 = Negate(x=w361) -> (-x=w363:dbl)
            n261 = Negate(x=w358) -> (-x=w360:dbl)
            n262 = Select(t=w363, s="Filp", f=w361) -> (s? t:f=w362:dbl)
            n263 = for {
              tunnel: w352 -> [w486] mode=indexing
              shift-right: [w482] -> w423
              shift-left: 0 -> [w481]
              tunnel: w358 -> [w485]
              i -> [w483]
              n264 = Greater?(x=w485, y=w486) -> (0:w484:bool)
              n265 = Select(t=w483, s=w484, f=w481) -> (s? t:f=w482:i32)
            }
            n266 = Select(t=w360, s="Filp", f=w358) -> (s? t:f=w359:dbl)
            n267 = property on="Grp_ExtVel_Hor" class="WFGraph (strict)"() -> ("CrsrList"=w415:T20)  [unwired: 2 in, 2 out]
            n268 = for {
              tunnel: w353 -> [_] mode=indexing
              tunnel: w364 -> [w489]
              tunnel: w362 -> [w488]
              tunnel: [w489] -> w434 mode=indexing
              tunnel: [w488] -> w433 mode=indexing
              tunnel: [w487] -> w425 mode=indexing
              tunnel: w359 -> [w487]
            }
            n269 = Negate(x=w352) -> (-x=w357:dbl[])
            n270 = Select(t=w357, s="Filp", f=w352) -> (s? t:f=w356:dbl[])
            n271 = Multiply(x=w372, y=w423) -> (x*y=w371:dbl)
            n272 = Bundle By Name("t0"=w419, "dt"=w372, "Y"=w356) -> (w417:waveform(dbl))  [unwired: 1 in]
            n273 = Bundle By Name("t0"=w419, "dt"=w372, "Y"=w434) -> (w435:waveform(dbl))  [unwired: 1 in]
            n274 = Bundle By Name("t0"=w419, "dt"=w372, "Y"=w433) -> (w432:waveform(dbl))  [unwired: 1 in]
            n275 = Bundle By Name("t0"=w419, "dt"=w372, "Y"=w425) -> (w426:waveform(dbl))  [unwired: 1 in]
            n276 = Multiply(x=w372, y=w373) -> (x*y=w370:dbl)
            n277 = Index Array(array=w415) -> (element #1=w414:T21, element #2=w375:T21)  [unwired: 2 in]
            n278 = Subtract(x=w371, y=w370) -> (x-y=→"Decaytime (Sec)":dbl)
            n279 = Unbundle(w414) -> ("Name"=w410:string, "Color"=w409:u32, "Style"=w408:u8, "Point Style"=w407:u8, "Name Visible"=w406:bool, "Allow Drag"=w405:bool, "Cursor Mode"=w404:u32, "Plot"=w403:i32, "Index"=w400:i32, "Position"=w412:cluster{"X":dbl, "Y":dbl}, "X Scale"=w401:u32, "Y Scale"=w399:u32, "Watch Plots"=w398:i32[], "Watch All Plots"=w397:bool, "Plot Area"=w396:i32, "Label Offset"=w395:cluster{"X":dbl, "Y":dbl})
            n280 = Unbundle(w375) -> ("Name"=w378:string, "Color"=w379:u32, "Style"=w380:u8, "Point Style"=w381:u8, "Name Visible"=w382:bool, "Allow Drag"=w383:bool, "Cursor Mode"=w384:u32, "Plot"=w385:i32, "Index"=w388:i32, "Position"=w376:cluster{"X":dbl, "Y":dbl}, "X Scale"=w387:u32, "Y Scale"=w389:u32, "Watch Plots"=w390:i32[], "Watch All Plots"=w391:bool, "Plot Area"=w392:i32, "Label Offset"=w393:cluster{"X":dbl, "Y":dbl})
            n281 = Build Array(w417, w438, w436, w435, w432, w426) -> (→"Grp_ExtVel_Hor":waveform(dbl)[])
            n282 = Unbundle By Name(w412) -> ("Y"=w411:dbl)
            n283 = Unbundle By Name(w376) -> ("Y"=w377:dbl)
            n284 = Bundle(w371, "Y"=w411) -> (w402:cluster{dbl, "Y":dbl})  [unwired: 1 in]
            n285 = Bundle(w370, "Y"=w377) -> (w386:cluster{dbl, "Y":dbl})  [unwired: 1 in]
            n286 = Bundle("Name"=w410, "Color"=w409, "Style"=w408, "Point Style"=w407, "Name Visible"=w406, "Allow Drag"=w405, "Cursor Mode"=w404, "Plot"=w403, "Index"=w400, w402, "X Scale"=w401, "Y Scale"=w399, "Watch Plots"=w398, "Watch All Plots"=w397, "Plot Area"=w396, "Label Offset"=w395) -> (w394:T22)  [unwired: 1 in]
            n287 = Bundle("Name"=w378, "Color"=w379, "Style"=w380, "Point Style"=w381, "Name Visible"=w382, "Allow Drag"=w383, "Cursor Mode"=w384, "Plot"=w385, "Index"=w388, w386, "X Scale"=w387, "Y Scale"=w389, "Watch Plots"=w390, "Watch All Plots"=w391, "Plot Area"=w392, "Label Offset"=w393) -> (w374:T22)  [unwired: 1 in]
            n288 = Build Array(w394, w374) -> (w413:T23)
            n289 = property on="Grp_ExtVel_Hor" class="WFGraph (strict)"("CrsrList"=w413) -> ()  [unwired: 2 in, 2 out]
          }
          frame "DetectMarker" {
            n290 = flat-sequence {
              tunnel: w501 -> [w521]
              frame #0 {
                w515 = 15.0 ("y")
                w527 = u16 0 items=["All", "Shift Information", "Rotation Information"] ("Learn Mode")
                n291 = property on="Img_Org" class="ImageControl"() -> ("ROI"=w519:T18)  [unwired: 2 in, 2 out]
                n292 = local read "BCGTD"() -> (w520:T8)
                n293 = Unbundle(w521) -> ("New Image"=w517:T9, "New Image"=w522:T9)  [unwired: 3 out]
                n294 = Unbundle(w520) -> ("Brightness"=w525:sgl, "Contrast"=w524:sgl, "Gamma"=w523:sgl, "Detection Sensitivity"=w516:sgl)
                n295 = Bundle("Brightness"=w525, "Contrast"=w524, "Gamma"=w523) -> ()  [unwired: 1 in, 1 out]
                n296 = Unbundle(w519) -> ("Global Rectangle"=w530:i32[])  [unwired: 1 out]
                n297 = call "IMAQ Extract"("Optional Rectangle"=w530, "Image Dst"=w522, "Image Src"=w517) -> ("error out"=w529:errorcluster, "Image Dst Out"=w526:T9)  [unwired: 3 in, 4 out]
                n298 = call "IMAQ Setup Learn Pattern 2"("Learn Mode"=w527) -> ("Learn Pattern Setup Data"=w528:string)  [unwired: 1 in, 9 out]
                n299 = call "IMAQ Learn Pattern 2"("error in (no error)"=w529, "Learn Pattern Setup Data"=w528, "Image"=w526) -> ("Template Image Out"=w518:T9)  [unwired: 1 in, 7 out]
                n300 = call "Dt_Marker.vi"("ROI Descriptor"=w519, "Minimum Match Score"=w516, "Img_Mrk"=w518, "Img_Mod"=w517) -> ("Position"=w506:cluster{"x":sgl, "y":sgl}, "Img_Mod_Out"=w507:T9, "x = 0?"=w503:bool)  [unwired: 3 in, 2 out]
                n301 = Unbundle(w506) -> ("x"=w505:sgl, "y"=w504:sgl)
                n302 = Not(x=w503) -> (.not. x?=w502:bool)
                n303 = property on="Marker Detection" class="Bool (strict)"("Value"=w502) -> ()  [unwired: 2 in, 2 out]
                n304 = Add(x=w505, y=w515) -> (x+y=w512:dbl)
                n305 = Add(x=w504, y=w515) -> (x+y=w511:dbl)
                n306 = Subtract(x=w505, y=w515) -> (x-y=w514:dbl)
                n307 = Subtract(x=w504, y=w515) -> (x-y=w513:dbl)
                n308 = Bundle(w514, w513, w512, w511) -> (w510:cluster{dbl, dbl, dbl, dbl})  [unwired: 1 in]
                n309 = call "IMAQ Overlay Oval"("Color"=u32 6618880, "Bounding Rectangle"=w510, "Image"=w507) -> ("Image Out"=w509:T9)  [unwired: 7 in, 1 out]
                n310 = local write "Img_Mod"(w509) -> ()
                n311 = local write "Img_Marker"(w518) -> ()
              }
              frame #1 {
                n312 = local read "FrameNum"() -> (w532:u32)
                n313 = property on="Img_Org" class="ImageControl"("ROI"=T18 {"Global Rectangle"=[], "Contours"=[]}) -> ()  [unwired: 2 in, 2 out]
                n314 = Equal To 0?(x=w532) -> (x = 0?=w531:bool)
                n315 = case shown="True" w531 {
                  frame False {
                  }
                  frame True {
                    n316 = property on="btn_Start" class="Bool"("DisabledEnum"=T19."Enabled" ("비활성화")) -> ()  [unwired: 2 in, 2 out]
                  }
                }
              }
            }
          }
          frame "FinalGrpOpen" {
            n317 = local read "Final Location: 2"() -> (w536:path)
            n318 = property on="Analyzed Data:" class="LstBox (strict)"() -> ("Item Names"=w544:string[])  [unwired: 2 in, 2 out]
            n319 = property on="Analyzed Data:" class="LstBox (strict)"() -> ("Value"=w539:i32)  [unwired: 2 in, 2 out]
            n320 = Not Equal?(x=w536, y=path "") -> (x != y?=w540:bool)
            n321 = Index Array(array=w544, index=w539) -> (element=w537:string)
            n322 = Not Equal?(x=w537, y="") -> (x != y?=w541:bool)
            n323 = And(x=w541, y=w540) -> (x .and. y?=w538:bool)
            n324 = case shown="True" w538 {
              tunnel: w537 -> [_ w548]
              tunnel: w536 -> [_ w547]
              tunnel: w535 -> [_ w568]
              frame False {
              }
              frame True {
                w565 = u32 0 ("Active Cursor")
                n325 = Search and Replace String(input string=w548, search string=".csv" ("검색 문자열"), replace string="_grph.csv" ("대체 문자열(\"\")")) -> (result string=w572:string)  [unwired: 5 in, 3 out]
                n326 = Search and Replace String(input string=w548, search string=".csv" ("검색 문자열"), replace string="_FitPara.csv" ("대체 문자열(\"\")")) -> (result string=w549:string)  [unwired: 5 in, 3 out]
                n327 = Build Path(base path=w547, name or relative path=w549) -> (appended path=w546:path)
                n328 = Build Path(base path=w547, name or relative path=w572) -> (appended path=w571:path)
                n329 = call-poly <vilib>:"Read From Spreadsheet File.vi"("delimiter (\\t)"="," ("delimiter (\\t)"), "file path (dialog if empty)"=w546) -> ("first row"=w561:dbl[])  [unwired: 5 in, 4 out]
                n330 = call <vilib>:"Read Waveform from File.vi"("file path (dialog if empty)"=w571) -> ("all waveforms in record"=w564:waveform(dbl)[])  [unwired: 5 in, 3 out]
                n331 = property on="Grp_Raw" class="WFGraph (strict)"("Value"=w564) -> (error out=w563:errorcluster)  [unwired: 2 in, 1 out]
                n332 = Index Array(array=w561) -> (element #1=w560:dbl, element #2=w559:dbl, element #3=w558:dbl, element #4=w557:dbl, element #5=w556:dbl, element #6=w555:dbl, element #7=w554:dbl, element #8=w553:dbl, element #9=w552:dbl)  [unwired: 9 in]
                n333 = Bundle(w560, w559, w558, w557, w556, w555, w554, w553, w552) -> (w545:T24)  [unwired: 1 in]
                n334 = property on="Grp_Raw" class="WFGraph (strict)"(error in=w563, "Active Cursor"=w565, "Cursor.Cursor Index"=w565, "Active Cursor"=u32 1) -> (error out=w566:errorcluster)  [unwired: 1 in, 1 out]
                n335 = Build Path(base path=w547, name or relative path=w548) -> (appended path=w570:path)
                n336 = property on="FittingParameter" class="Clust (strict)"("Value"=w545) -> ()  [unwired: 2 in, 2 out]
                n337 = Enqueue Element(queue=w568, element=T17."SelPlot" ("Enum"), error in (no error)=w566) -> ()  [unwired: 1 in, 3 out]
                n338 = disable-structure shown="Disabled" {
                  disable-tunnel: w570 -> [w587 _]
                  frame Disabled {
                    w581 = 0 ("인덱스 (행)")
                    n339 = call-poly <vilib>:"Read From Spreadsheet File.vi"("delimiter (\\t)"="," ("delimiter (\\t)"), "format (%.3f)"="%.6f", "file path (dialog if empty)"=w587) -> ("all rows"=w578:dbl[][])  [unwired: 4 in, 4 out]
                    n340 = Index Array(array=w578, index (row) #1=w581, index (col) #1=2 ("인덱스 (행)"), index (row) #2=w581, index (col) #2=w581, index (row) #3=w581, index (col) #3=1 ("인덱스 (행)")) -> (element #1=w579:dbl, element #2=w584:dbl, element #3=w583:dbl)
                    n341 = Delete From Array(array=w578, index (row)=0 ("인덱스 (행)")) -> (array with subset deleted=w576:dbl[][])  [unwired: 2 in, 1 out]
                    n342 = property on="#Cycles" class="DigNum (strict)"("Value"=w579) -> ()  [unwired: 2 in, 2 out]
                    n343 = Number To Fractional String(number=w576) -> (F-format string=w575:string[][])  [unwired: 3 in]
                    n344 = property on="period" class="DigNum (strict)"("Value"=w584) -> ()  [unwired: 2 in, 2 out]
                    n345 = property on="AMHV" class="DigNum (strict)"("Value"=w583) -> ()  [unwired: 2 in, 2 out]
                    n346 = property on="Table" class="Tbl (strict)"("Value"=w575) -> ()  [unwired: 2 in, 2 out]
                  }
                  frame Enabled {
                  }
                }
              }
            }
          }
          frame "RmvGrp" {
            n347 = local read "RawTemp"() -> (w588:waveform(dbl)[][])
            n348 = property on="Grp_Raw" class="WFGraph (strict)"("Active Cursor"=u32 0, "Active Cursor"=u32 1, "Active Cursor"=u32 2) -> ("Cursor.Cursor Index"=w599:i32, "Cursor.Cursor Index"=w598:i32, "Value"=w590:waveform(dbl)[], "Cursor.Cursor Index"=w591:i32)  [unwired: 2 in, 2 out]
            n349 = Max & Min(x=w599, y=w598) -> (max(x,y)=w597:i32, min(x,y)=w596:i32)
            n350 = Build Array (concatenate)(w588, w590) -> (→"RawTemp":waveform(dbl)[][])
            n351 = Subtract(x=w597, y=w596) -> (x-y=w595:i32)
            n352 = case shown="True" "Point Removal" {
              tunnel: w590 -> [w619 w643]
              tunnel: w596 -> [w612 _]
              tunnel: w595 -> [w611 _]
              tunnel: [w602 w650] -> w594
              tunnel: w591 -> [_ w642]
              frame False {
                n353 = call "다이나믹 데이터로부터 변환11"("Dynamic Data Type"=w619) -> ("Waveform"=w614:waveform(dbl))  [unwired: 3 in]
                n354 = call "다이나믹 데이터로부터 변환12"("Dynamic Data Type"=w619) -> ("Waveform"=w613:waveform(dbl))  [unwired: 3 in]
                n355 = call "다이나믹 데이터로부터 변환9"("Dynamic Data Type"=w619) -> ("Waveform"=w616:waveform(dbl))  [unwired: 3 in]
                n356 = call "다이나믹 데이터로부터 변환10"("Dynamic Data Type"=w619) -> ("Waveform"=w615:waveform(dbl))  [unwired: 3 in]
                n357 = call "다이나믹 데이터로부터 변환5"("Dynamic Data Type"=w619) -> ("Waveform"=w637:waveform(dbl))  [unwired: 3 in]
                n358 = call "다이나믹 데이터로부터 변환6"("Dynamic Data Type"=w619) -> ("Waveform"=w632:waveform(dbl))  [unwired: 3 in]
                n359 = call "다이나믹 데이터로부터 변환7"("Dynamic Data Type"=w619) -> ("Waveform"=w618:waveform(dbl))  [unwired: 3 in]
                n360 = call "다이나믹 데이터로부터 변환8"("Dynamic Data Type"=w619) -> ("Waveform"=w617:waveform(dbl))  [unwired: 3 in]
                n361 = Unbundle By Name(w614) -> ("Y"=w623:dbl[])
                n362 = Unbundle By Name(w613) -> ("Y"=w620:dbl[])
                n363 = Unbundle By Name(w616) -> ("Y"=w627:dbl[])
                n364 = Unbundle By Name(w615) -> ("Y"=w624:dbl[])
                n365 = Unbundle By Name(w637) -> ("Y"=w636:dbl[])
                n366 = Unbundle By Name(w632) -> ("Y"=w633:dbl[])
                n367 = Unbundle By Name(w618) -> ("Y"=w631:dbl[])
                n368 = Unbundle By Name(w617) -> ("Y"=w628:dbl[])
                n369 = Delete From Array(array=w623, length=w611, index=w612) -> (array with subset deleted=w622:dbl[])  [unwired: 1 out]
                n370 = Delete From Array(array=w620, length=w611, index=w612) -> (array with subset deleted=w621:dbl[])  [unwired: 1 out]
                n371 = Delete From Array(array=w627, length=w611, index=w612) -> (array with subset deleted=w626:dbl[])  [unwired: 1 out]
                n372 = Delete From Array(array=w624, length=w611, index=w612) -> (array with subset deleted=w625:dbl[])  [unwired: 1 out]
                n373 = Delete From Array(array=w636, length=w611, index=w612) -> (array with subset deleted=w635:dbl[])  [unwired: 1 out]
                n374 = Delete From Array(array=w633, length=w611, index=w612) -> (array with subset deleted=w634:dbl[])  [unwired: 1 out]
                n375 = Delete From Array(array=w631, length=w611, index=w612) -> (array with subset deleted=w630:dbl[])  [unwired: 1 out]
                n376 = Delete From Array(array=w628, length=w611, index=w612) -> (array with subset deleted=w629:dbl[])  [unwired: 1 out]
                n377 = Bundle By Name(cluster=w614, "Y"=w622) -> (w604:waveform(dbl))
                n378 = Bundle By Name(cluster=w613, "Y"=w621) -> (w603:waveform(dbl))
                n379 = Bundle By Name(cluster=w616, "Y"=w626) -> (w606:waveform(dbl))
                n380 = Bundle By Name(cluster=w615, "Y"=w625) -> (w605:waveform(dbl))
                n381 = Bundle By Name(cluster=w637, "Y"=w635) -> (w610:waveform(dbl))
                n382 = Bundle By Name(cluster=w632, "Y"=w634) -> (w609:waveform(dbl))
                n383 = Bundle By Name(cluster=w618, "Y"=w630) -> (w608:waveform(dbl))
                n384 = Bundle By Name(cluster=w617, "Y"=w629) -> (w607:waveform(dbl))
                n385 = Merge Signals(w610, w609, w608, w607, w606, w605, w604, w603) -> (w602:dynamicdata)
              }
              frame True {
                n386 = call "다이나믹 데이터로부터 변환16"("Dynamic Data Type"=w643) -> ("Waveform"=w644:waveform(dbl))  [unwired: 3 in]
                n387 = call "다이나믹 데이터로부터 변환2"("Dynamic Data Type"=w643) -> ("Waveform"=w648:waveform(dbl))  [unwired: 3 in]
                n388 = call "다이나믹 데이터로부터 변환4"("Dynamic Data Type"=w643) -> ("Waveform"=w647:waveform(dbl))  [unwired: 3 in]
                n389 = call "다이나믹 데이터로부터 변환14"("Dynamic Data Type"=w643) -> ("Waveform"=w646:waveform(dbl))  [unwired: 3 in]
                n390 = call "다이나믹 데이터로부터 변환15"("Dynamic Data Type"=w643) -> ("Waveform"=w645:waveform(dbl))  [unwired: 3 in]
                n391 = case shown="7" "Ring" {
                  tunnel: w643 -> [w658 w669 w680]
                  tunnel: w643 -> [w657 w668 w679]
                  tunnel: w643 -> [w656 w667 w678]
                  tunnel: w642 -> [w655 w666 w675]
                  tunnel: 0 ("length") -> [w654 w665 w674]
                  tunnel: [w653 w662 w677] -> w640
                  tunnel: [w652 w663 w676] -> w639
                  tunnel: [w651 w664 w673] -> w638
                  frame 5, Default {
                    n392 = call "다이나믹 데이터로부터 변환18"("Dynamic Data Type"=w657) -> ("Waveform"=w652:waveform(dbl))  [unwired: 3 in]
                    n393 = call "다이나믹 데이터로부터 변환19"("Dynamic Data Type"=w656) -> ("Waveform"=w651:waveform(dbl))  [unwired: 3 in]
                    n394 = call "다이나믹 데이터로부터 변환17"("Dynamic Data Type"=w658) -> ("Waveform"=w661:waveform(dbl))  [unwired: 3 in]
                    n395 = Unbundle By Name(w661) -> ("Y"=w660:dbl[])
                    n396 = Replace Array Subset(array=w660, new element=w654, index=w655) -> (w659:dbl[])
                    n397 = Bundle By Name(cluster=w661, "Y"=w659) -> (w653:waveform(dbl))
                  }
                  frame 6 {
                    n398 = call "다이나믹 데이터로부터 변환21"("Dynamic Data Type"=w668) -> ("Waveform"=w672:waveform(dbl))  [unwired: 3 in]
                    n399 = call "다이나믹 데이터로부터 변환22"("Dynamic Data Type"=w667) -> ("Waveform"=w664:waveform(dbl))  [unwired: 3 in]
                    n400 = call "다이나믹 데이터로부터 변환20"("Dynamic Data Type"=w669) -> ("Waveform"=w662:waveform(dbl))  [unwired: 3 in]
                    n401 = Unbundle By Name(w672) -> ("Y"=w670:dbl[])
                    n402 = Replace Array Subset(array=w670, new element=w665, index=w666) -> (w671:dbl[])
                    n403 = Bundle By Name(cluster=w672, "Y"=w671) -> (w663:waveform(dbl))
                  }
                  frame 7 {
                    n404 = call "다이나믹 데이터로부터 변환24"("Dynamic Data Type"=w679) -> ("Waveform"=w676:waveform(dbl))  [unwired: 3 in]
                    n405 = call "다이나믹 데이터로부터 변환25"("Dynamic Data Type"=w678) -> ("Waveform"=w683:waveform(dbl))  [unwired: 3 in]
                    n406 = call "다이나믹 데이터로부터 변환23"("Dynamic Data Type"=w680) -> ("Waveform"=w677:waveform(dbl))  [unwired: 3 in]
                    n407 = Unbundle By Name(w683) -> ("Y"=w682:dbl[])
                    n408 = Replace Array Subset(array=w682, new element=w674, index=w675) -> (w681:dbl[])
                    n409 = Bundle By Name(cluster=w683, "Y"=w681) -> (w673:waveform(dbl))
                  }
                }
                n410 = Merge Signals(w648, w647, w646, w645, w644, w640, w639, w638) -> (w650:dynamicdata)
              }
            }
            n411 = property on="Grp_Raw" class="WFGraph (strict)"("Value"=w594) -> ()  [unwired: 2 in, 2 out]
          }
          frame "SaveAnResult" {
            w689 = T16 0 items=["no dialog", "OK message", "continue or stop message", "OK message + warnings", "continue/stop + warnings"] ("type of dialog (OK msg:1)")
            n412 = property on="Raw Location:" class="Path"() -> ("Value"=w686:path)  [unwired: 2 in, 2 out]
            n413 = call "File Dialog"("start path"=w686, "pattern (all files)"="*.csv") -> ("selected path"=w684:path, "cancelled"=w685:bool, "error out"=w688:errorcluster)  [unwired: 10 in, 1 out]
            n414 = call <vilib>:"General Error Handler.vi"("type of dialog (OK msg:1)"=w689, "error in (no error)"=w688) -> ()  [unwired: 9 in, 5 out]
            n415 = case shown="False" w685 {
              tunnel: w684 -> [w751 _]
              frame False {
                n416 = Strip Path(path=w751) -> (stripped path=w750:path, name=w713:string)
                n417 = Build Path(base path=w750, name or relative path="GrpImgs" ("검색 문자열")) -> (appended path=w748:path)
                n418 = case shown="False" "Img_Only" {
                  tunnel: w751 -> [w761 _]
                  frame False {
                    (unwired) "," ("delimiter (\\t)")
                    n419 = Strip Path(path=w761) -> (stripped path=w766:path, name=w765:string)
                    n420 = Strip Path(path=w761) -> (stripped path=w807:path, name=w806:string)
                    n421 = property on="Grp_ExtPos" class="WFGraph (strict)"() -> ("Value"=w792:waveform(dbl)[])  [unwired: 2 in, 2 out]
                    n422 = property on="Grp_ExtVel" class="WFGraph (strict)"() -> ("Value"=w791:waveform(dbl)[])  [unwired: 2 in, 2 out]
                    n423 = Search and Replace String(input string=w765, search string=".csv" ("검색 문자열"), replace string="_DecayTime.csv" ("대체 문자열(\"\")")) -> (result string=w762:string)  [unwired: 5 in, 3 out]
                    n424 = Search and Replace String(input string=w806, search string=".csv" ("검색 문자열"), replace string="_grph.csv" ("대체 문자열(\"\")")) -> (result string=w803:string)  [unwired: 5 in, 3 out]
                    n425 = Build Path(base path=w766, name or relative path=w762) -> (appended path=w759:path)
                    n426 = Build Path(base path=w807, name or relative path=w803) -> (appended path=w802:path)
                    n427 = Strip Path(path=w761) -> (stripped path=w796:path, name=w797:string)
                    n428 = local read "Decaytime (Sec)"() -> (w758:dbl)
                    n429 = Search and Replace String(input string=w797, search string=".csv" ("검색 문자열"), replace string="_FitPara.csv" ("대체 문자열(\"\")")) -> (result string=w800:string)  [unwired: 5 in, 3 out]
                    n430 = Build Array (concatenate)(w792, w791) -> (w790:waveform(dbl)[])
                    n431 = Build Path(base path=w796, name or relative path=w800) -> (appended path=w768:path)
                    n432 = call-poly <vilib>:"Write Waveforms to File.vi"("waveform array"=w790, "file path (dialog if empty)"=w802) -> ()  [unwired: 8 in, 2 out]
                    n433 = Number To Fractional String(number=w758) -> (F-format string=w757:string)  [unwired: 3 in]
                    n434 = property on="period" class="DigNum (strict)"() -> ("Value"=w811:dbl)  [unwired: 2 in, 2 out]
                    n435 = property on="AMHV" class="DigNum (strict)"() -> ("Value"=w810:dbl)  [unwired: 2 in, 2 out]
                    n436 = property on="#Cycles" class="DigNum (strict)"() -> ("Value"=w801:dbl)  [unwired: 2 in, 2 out]
                    n437 = Build Array(w757) -> (w756:string[])
                    n438 = property on="Table" class="Tbl (strict)"() -> ("Column Headers[]"=w789:string[])  [unwired: 2 in, 2 out]
                    n439 = property on="Table" class="Tbl (strict)"() -> ("Value"=w787:string[][])  [unwired: 2 in, 2 out]
                    n440 = Build Array(w811, w810, w801) -> (w795:dbl[])
                    n441 = call-poly <vilib>:"Write To Spreadsheet File.vi"("delimiter (\\t)"="," ("delimiter (\\t)"), "1D data"=w756, "file path (dialog if empty)"=w759) -> ()  [unwired: 5 in, 1 out]
                    n442 = Number To Fractional String(number=w795, precision (6)=i16 6 ("정밀도(6)")) -> (F-format string=w794:string[])  [unwired: 2 in]
                    n443 = Insert Into Array(array=w787, index (row)=0 ("disabled index (col)"), new element=w789) -> (w785:string[][])  [unwired: 1 in]
                    n444 = property on="FittingParameter" class="Clust (strict)"() -> ("Value"=w767:T1)  [unwired: 2 in, 2 out]
                    n445 = property on="Table" class="Tbl (strict)"() -> ("Row Headers[]"=w783:string[])  [unwired: 2 in, 2 out]
                    n446 = Insert Into Array(array=w783, index=0, new element="" ("new element/subarray")) -> (w782:string[])
                    n447 = Insert Into Array(array=w785, index (col)=0 ("disabled index (col)"), new element=w782) -> (w784:string[][])  [unwired: 1 in]
                    n448 = Build Array (concatenate)(w794, w784) -> (w809:string[][])
                    n449 = call-poly <vilib>:"Write To Spreadsheet File.vi"("delimiter (\\t)"="," ("delimiter (\\t)"), "2D data"=w809, "file path (dialog if empty)"=w761) -> ()  [unwired: 5 in, 1 out]
                    n450 = Unbundle By Name(w767) -> ("HorL_Threshold"=w779:dbl, "HorR_Threshold"=w778:dbl, "HorPk Width"=w777:i32, "VerL_Threshold"=w776:dbl, "VerR_Threshold"=w775:dbl, "VerPk Width"=w774:i32, "TorL_Threshold 3"=w773:dbl, "TorR_Threshold"=w772:dbl, "TorPk Width 3"=w771:i32)
                    n451 = Build Array(w779, w778, w777, w776, w775, w774, w773, w772, w771) -> (w770:dbl[])
                    n452 = call-poly <vilib>:"Write To Spreadsheet File.vi"("delimiter (\\t)"="," ("delimiter (\\t)"), "1D data"=w770, "file path (dialog if empty)"=w768) -> ()  [unwired: 5 in, 1 out]
                  }
                  frame True {
                  }
                }
                n453 = call <vilib>:"Check if File or Folder Exists.vi"("path"=w748) -> ("file or folder exists?"=w747:bool, "dup path"=w712:path)  [unwired: 8 in, 1 out]
                n454 = case shown="True" w747 {
                  tunnel: w712 -> [w754 w755]
                  tunnel: [w753 w755] -> w746
                  frame False {
                    n455 = Create Folder(path (use dialog)=w754) -> (created path=w753:path)  [unwired: 2 in, 2 out]
                  }
                  frame True {
                  }
                }
                n456 = Search and Replace String(input string=w713, search string=".csv" ("검색 문자열"), replace string="_Pos.bmp" ("대체 문자열(\"\")")) -> (result string=w741:string)  [unwired: 5 in, 3 out]
                n457 = Search and Replace String(input string=w713, search string=".csv" ("검색 문자열"), replace string="_CycVer.bmp" ("대체 문자열(\"\")")) -> (result string=w725:string)  [unwired: 5 in, 3 out]
                n458 = Search and Replace String(input string=w713, search string=".csv" ("검색 문자열"), replace string="_VelTor.bmp" ("대체 문자열(\"\")")) -> (result string=w729:string)  [unwired: 5 in, 3 out]
                n459 = Search and Replace String(input string=w713, search string=".csv" ("검색 문자열"), replace string="_VelHor.bmp" ("대체 문자열(\"\")")) -> (result string=w733:string)  [unwired: 5 in, 3 out]
                n460 = Build Path(base path=w712, name or relative path=w741) -> (appended path=w738:path)
                n461 = Build Path(base path=w712, name or relative path=w725) -> (appended path=w720:path)
                n462 = Build Path(base path=w712, name or relative path=w729) -> (appended path=w721:path)
                n463 = Build Path(base path=w712, name or relative path=w733) -> (appended path=w722:path)
                n464 = invoke on="Grp_CycleAnal_Ver" class="WFGraph (strict)" method="Export Image"("FileType"=enum32{"BMP", "EPS", "EMF", "PICT"}."BMP" ("File Type"), "Target"=enum32{"File", "Clipboard"}."File", "Path"=w720) -> ()  [unwired: 5 in, 8 out]
                n465 = invoke on="Grp_ExtPos" class="WFGraph (strict)" method="Export Image"("FileType"=enum32{"BMP", "EPS", "EMF", "PICT"}."BMP" ("File Type"), "Target"=enum32{"File", "Clipboard"}."File", "Path"=w738) -> ()  [unwired: 5 in, 8 out]
                n466 = invoke on="Grp_ExtVel_Hor" class="WFGraph (strict)" method="Export Image"("FileType"=enum32{"BMP", "EPS", "EMF", "PICT"}."BMP" ("File Type"), "Target"=enum32{"File", "Clipboard"}."File", "Path"=w722) -> ()  [unwired: 5 in, 8 out]
                n467 = invoke on="Grp_ExtVel_Tor" class="WFGraph (strict)" method="Export Image"("FileType"=enum32{"BMP", "EPS", "EMF", "PICT"}."BMP" ("File Type"), "Target"=enum32{"File", "Clipboard"}."File", "Path"=w721) -> ()  [unwired: 5 in, 8 out]
                n468 = Search and Replace String(input string=w713, search string=".csv" ("검색 문자열"), replace string="_Raw.bmp" ("대체 문자열(\"\")")) -> (result string=w743:string)  [unwired: 5 in, 3 out]
                n469 = Build Path(base path=w746, name or relative path=w743) -> (appended path=w742:path)
                n470 = invoke on="Grp_Raw" class="WFGraph (strict)" method="Export Image"("FileType"=enum32{"BMP", "EPS", "EMF", "PICT"}."BMP" ("File Type"), "Target"=enum32{"File", "Clipboard"}."File", "Path"=w742) -> ()  [unwired: 5 in, 8 out]
                n471 = Search and Replace String(input string=w713, search string=".csv" ("검색 문자열"), replace string="_Vel.bmp" ("대체 문자열(\"\")")) -> (result string=w735:string)  [unwired: 5 in, 3 out]
                n472 = Search and Replace String(input string=w713, search string=".csv" ("검색 문자열"), replace string="_CycTor.bmp" ("대체 문자열(\"\")")) -> (result string=w724:string)  [unwired: 5 in, 3 out]
                n473 = Search and Replace String(input string=w713, search string=".csv" ("검색 문자열"), replace string="_CycHor.bmp" ("대체 문자열(\"\")")) -> (result string=w728:string)  [unwired: 5 in, 3 out]
                n474 = Search and Replace String(input string=w713, search string=".csv" ("검색 문자열"), replace string="_VelVer.bmp" ("대체 문자열(\"\")")) -> (result string=w732:string)  [unwired: 5 in, 3 out]
                n475 = Build Path(base path=w712, name or relative path=w735) -> (appended path=w708:path)
                n476 = Build Path(base path=w712, name or relative path=w724) -> (appended path=w711:path)
                n477 = Build Path(base path=w712, name or relative path=w728) -> (appended path=w710:path)
                n478 = Build Path(base path=w712, name or relative path=w732) -> (appended path=w709:path)
                n479 = invoke on="Grp_CycleAnal_Tor" class="WFGraph (strict)" method="Export Image"("FileType"=enum32{"BMP", "EPS", "EMF", "PICT"}."BMP" ("File Type"), "Target"=enum32{"File", "Clipboard"}."File", "Path"=w711) -> ()  [unwired: 5 in, 8 out]
                n480 = invoke on="Grp_ExtVel" class="WFGraph (strict)" method="Export Image"("FileType"=enum32{"BMP", "EPS", "EMF", "PICT"}."BMP" ("File Type"), "Target"=enum32{"File", "Clipboard"}."File", "Path"=w708) -> ()  [unwired: 5 in, 8 out]
                n481 = invoke on="Grp_ExtVel_Ver" class="WFGraph (strict)" method="Export Image"("FileType"=enum32{"BMP", "EPS", "EMF", "PICT"}."BMP" ("File Type"), "Target"=enum32{"File", "Clipboard"}."File", "Path"=w709) -> ()  [unwired: 5 in, 8 out]
                n482 = invoke on="Grp_CycleAnal_Hor" class="WFGraph (strict)" method="Export Image"("FileType"=enum32{"BMP", "EPS", "EMF", "PICT"}."BMP" ("File Type"), "Target"=enum32{"File", "Clipboard"}."File", "Path"=w710) -> ()  [unwired: 5 in, 8 out]
              }
              frame True {
              }
            }
          }
          frame "Undo" {
            n483 = local read "RawTemp"() -> (w815:waveform(dbl)[][])
            n484 = Array Size(array=w815) -> (size(s)=w817:i32[])
            n485 = Index Array(array=w817, index=0) -> (element=w814:i32)
            n486 = Greater Than 0?(x=w814) -> (x > 0?=w812:bool)
            n487 = Not(x=w812) -> (.not. x?=→"x > 0?":bool)
            n488 = case shown="True" w812 {
              tunnel: w815 -> [_ w821]
              tunnel: w814 -> [_ w822]
              frame False {
              }
              frame True {
                n489 = Decrement(x=w822) -> (x-1=w820:i32)
                n490 = Delete From Array(array=w821, index (row)=w820) -> (deleted portion=w818:waveform(dbl)[], array with subset deleted=w819:waveform(dbl)[][])  [unwired: 2 in]
                n491 = local write "RawTemp"(w819) -> ()
                n492 = property on="Grp_Raw" class="WFGraph (strict)"("Value"=w818) -> ()  [unwired: 2 in, 2 out]
              }
            }
          }
        }
      }
      frame Error {
      }
    }
  }
  n493 = while {
    shift-right: [w833] -> w20
    shift-left: w19 -> [w836]
    tunnel: w21 -> [w837]
    shift-right: [w827] -> w15
    shift-left: w17 -> [w831]
    tunnel: w3 -> [w832]
    tunnel: w4 -> [w830]
    shift-right: [w825] -> w14
    shift-left: w16 -> [w829]
    stop <- w834 stop-if-true
    n494 = event shown="[14] \"Grp_Raw\": Cursor Move;  \"index\", \"# of terms\": Value Change" {
      selector: _ -> [_ _ _ _ _ _ _ _ _ _ _ _ _ _ _ _ _ _ _ _ _ _ _ _ _ _ _ _ _ _ _ _ _ _]
      dyn-events: _ -> [_ _ _ _ _ _ _ _ _ _ _ _ _ _ _ _ _ _ _ _ _ _ _ _ _ _ _ _ _ _ _ _ _ _]
      timeout: _ -> [_ _ _ _ _ _ _ _ _ _ _ _ _ _ _ _ _ _ _ _ _ _ _ _ _ _ _ _ _ _ _ _ _ _]
      tunnel: w837 -> [w841 w845 w849 w853 _ w861 w864 _ _ _ _ _ _ _ _ _ _ _ _ _ _ _ _ _ _ _ _ _ _ _ _ _ _ _]
      tunnel: w836 -> [w840 w844 w848 w851 _ w860 w863 _ _ _ _ _ _ _ _ _ _ _ _ _ _ _ _ _ _ _ _ _ _ _ _ _ w987 _]
      tunnel: [w839 w843 w847 w852 _ w859 w865 _ _ _ _ _ _ _ _ _ _ _ _ _ _ _ _ w953 _ _ _ _ _ _ _ _ w987 _] -> w833
      tunnel: [_ _ _ _ _ _ _ _ _ _ _ _ _ _ _ _ _ _ _ _ _ _ _ _ _ _ _ _ _ _ _ _ "Close" _] -> w835
      tunnel: w832 -> [_ _ _ _ w855 _ _ w869 w872 w876 w880 w883 w887 w892 _ w912 w916 w920 w932 _ _ _ _ _ _ _ _ _ _ _ _ _ _ _]
      tunnel: w831 -> [_ _ _ _ w857 _ _ w868 w873 w877 w881 w885 w888 w893 _ w913 w915 w919 w933 _ _ _ _ _ _ _ _ _ _ _ _ _ w985 _]
      tunnel: w830 -> [_ _ _ _ _ _ _ _ _ _ _ _ _ _ _ _ _ _ _ w937 w941 w945 w949 w952 _ w958 w961 w966 w971 w975 w979 w983 _ _]
      tunnel: w829 -> [_ _ _ _ _ _ _ _ _ _ _ _ _ _ _ _ _ _ _ w936 w940 w944 w948 w951 _ w957 w962 w965 w970 w974 w978 w982 w984 _]
      tunnel: [_ _ _ _ w856 _ _ w867 w871 w875 w879 w884 w889 w891 _ w911 w914 w918 w931 _ _ _ _ _ _ _ _ _ _ _ _ _ w985 _] -> w827
      tunnel: [_ _ _ _ _ _ _ _ _ _ _ _ _ _ _ _ _ _ _ w934 w938 w943 w947 _ _ w959 w963 w967 w969 w973 w977 w981 w984 _] -> w825
      event "Video File": Value Change {
        n495 = event-data() -> ()  [unwired: 1 in, 1 out]
        n496 = Enqueue Element(queue=w841, element=T13."VideoFileOpen" ("Enum"), error in (no error)=w840) -> (error out=w839:errorcluster)  [unwired: 1 in, 2 out]
      }
      event "CalVar_VA": Value Change {
        n497 = event-data() -> ()  [unwired: 1 in, 1 out]
        n498 = Enqueue Element(queue=w845, element=T13."CalvarOpen" ("Enum"), error in (no error)=w844) -> (error out=w843:errorcluster)  [unwired: 1 in, 2 out]
      }
      event "Cal_Val:": Value Change {
        n499 = event-data() -> ()  [unwired: 1 in, 1 out]
        n500 = Enqueue Element(queue=w849, element=T13."CalDateChange" ("Enum"), error in (no error)=w848) -> (error out=w847:errorcluster)  [unwired: 1 in, 2 out]
      }
      event "BCGTD", "Marker Edge 1", "Marker Edge 2", "Marker Edge 3": Value Change {
        n501 = event-data() -> ()  [unwired: 1 in, 1 out]
        n502 = Enqueue Element(queue=w853, element=T13."Adj_BCGTD" ("Enum"), error in (no error)=w851) -> (error out=w852:errorcluster)  [unwired: 1 in, 2 out]
      }
      event "btn_Detect": Value Change {
        n503 = event-data() -> ()  [unwired: 1 in, 1 out]
        n504 = Enqueue Element(queue=w855, element=T25."DetectMarker" ("Enum"), error in (no error)=w857) -> (error out=w856:errorcluster)  [unwired: 1 in, 2 out]
      }
      event "btn_Start": Value Change {
        n505 = event-data() -> ()  [unwired: 1 in, 1 out]
        n506 = Enqueue Element(queue=w861, element=T13."StartTrack" ("Enum"), error in (no error)=w860) -> (error out=w859:errorcluster)  [unwired: 1 in, 2 out]
      }
      event "btn_SaveResult": Value Change {
        n507 = event-data() -> ()  [unwired: 1 in, 1 out]
        n508 = Enqueue Element(queue=w864, element=T13."SaveResult" ("Enum"), error in (no error)=w863) -> (error out=w865:errorcluster)  [unwired: 1 in, 2 out]
      }
      event "Raw Location:": Value Change {
        n509 = event-data() -> ()  [unwired: 1 in, 1 out]
        n510 = Enqueue Element(queue=w869, element=T17."RawDataOpen" ("Enum"), error in (no error)=w868) -> (error out=w867:errorcluster)  [unwired: 1 in, 2 out]
      }
      event "Final Location: 2": Value Change {
        n511 = event-data() -> ()  [unwired: 1 in, 1 out]
        n512 = Enqueue Element(queue=w872, element=T17."FinalDataOpen" ("Enum"), error in (no error)=w873) -> (error out=w871:errorcluster)  [unwired: 1 in, 2 out]
      }
      event "CalVar_GA": Value Change {
        n513 = event-data() -> ()  [unwired: 1 in, 1 out]
        n514 = Enqueue Element(queue=w876, element=T17."Calvar2Open" ("Enum"), error in (no error)=w877) -> (error out=w875:errorcluster)  [unwired: 1 in, 2 out]
      }
      event "Cal_Val: 2": Value Change {
        n515 = event-data() -> ()  [unwired: 1 in, 1 out]
        n516 = Enqueue Element(queue=w880, element=T17."Cal2DateChange" ("Enum"), error in (no error)=w881) -> (error out=w879:errorcluster)  [unwired: 1 in, 2 out]
      }
      event "Raw Data:": Double Click {
        n517 = event-data() -> ()  [unwired: 1 in, 4 out]
        n518 = Enqueue Element(queue=w883, element=T17."RawGrpOpen" ("Enum"), error in (no error)=w885) -> (error out=w884:errorcluster)  [unwired: 1 in, 2 out]
      }
      event "Analyzed Data:": Double Click {
        n519 = event-data() -> ()  [unwired: 1 in, 1 out]
        n520 = Enqueue Element(queue=w887, element=T17."FinalGrpOpen" ("Enum"), error in (no error)=w888) -> (error out=w889:errorcluster)  [unwired: 1 in, 2 out]
      }
      event "Grp_Raw": Cursor Release; "btn_Analyze", "HorR_Threshold", "HorL_Threshold", "HorPk Width", "VerPk Width", "VerR_Threshold", "VerL_Threshold", "TorPk Width 3", "TorR_Threshold", "TorL_Threshold", "filterRank", "filterRank 2", "Filp", "Enum": Value Change {
        n521 = event-data() -> ()  [unwired: 1 in, 2 out]
        n522 = case shown="True" "btn_Analyze" {
          tunnel: w893 -> [w894 w898]
          tunnel: w892 -> [_ w897]
          tunnel: [w894 w896] -> w891
          frame False {
          }
          frame True {
            n523 = Enqueue Element(queue=w897, element=T17."SelGrp" ("Enum"), error in (no error)=w898) -> (error out=w896:errorcluster)  [unwired: 1 in, 2 out]
          }
        }
      }
      event "Grp_Raw": Cursor Move; "index", "# of terms": Value Change {
        n524 = event-data() -> ()  [unwired: 1 in, 2 out]
        n525 = local read "index"() -> (w899:i32)
        n526 = local read "Grp_Raw"() -> (w900:waveform(dbl)[])
        n527 = local read "# of terms"() -> (w908:i32)
        n528 = property on="Grp_Raw" class="WFGraph (strict)"() -> ("CrsrList"=w909:T20)  [unwired: 2 in, 2 out]
        n529 = Subtract(x=w899, y=1) -> (x-y=w903:i32)
        n530 = Index Array(array=w900, index=w903) -> (element=w901:waveform(dbl))
        n531 = call "signalProcessing.vi"("number of terms"=w908, "array"=w909, "waveform in"=w901) -> ("Frequencies"=w904:dbl[], "output waveform"=w906:waveform(dbl))  [unwired: 6 in, 1 out]
        n532 = local write "Frequencies"(w904) -> ()
        n533 = Replace Array Subset(array=w900, new element=w906, index=8) -> (w905:waveform(dbl)[])
        n534 = local write "Grp_Raw"(w905) -> ()
      }
      event "btn_Remove": Value Change {
        n535 = event-data() -> ()  [unwired: 1 in, 1 out]
        n536 = Enqueue Element(queue=w912, element=T17."RmvGrp" ("Enum"), error in (no error)=w913) -> (error out=w911:errorcluster)  [unwired: 1 in, 2 out]
      }
      event "btn_Undo": Value Change {
        n537 = event-data() -> ()  [unwired: 1 in, 1 out]
        n538 = Enqueue Element(queue=w916, element=T11."Undo" ("Enum"), error in (no error)=w915) -> (error out=w914:errorcluster)  [unwired: 1 in, 2 out]
      }
      event "Filter Intensity": Value Change {
        n539 = event-data() -> ()  [unwired: 1 in, 1 out]
        n540 = property on="Grp_Raw" class="WFGraph (strict)"() -> ("Value"=w922:waveform(dbl)[])  [unwired: 2 in, 2 out]
        n541 = call "다이나믹 데이터로부터 변환"("Dynamic Data Type"=w922) -> ("Array"=w923:dbl[])  [unwired: 3 in]
        n542 = Empty Array?(array=w923) -> (empty?=w924:bool)
        n543 = Not(x=w924) -> (.not. x?=w921:bool)
        n544 = case shown="True" w921 {
          tunnel: w920 -> [_ w928]
          tunnel: w919 -> [w925 w927]
          tunnel: [w925 w926] -> w918
          frame False {
          }
          frame True {
            n545 = Enqueue Element(queue=w928, element=T17."SelGrp" ("Enum"), error in (no error)=w927) -> (error out=w926:errorcluster)  [unwired: 1 in, 2 out]
          }
        }
      }
      event "btn_SaveAnResult": Value Change {
        n546 = event-data() -> ()  [unwired: 1 in, 1 out]
        n547 = Enqueue Element(queue=w932, element=T17."SaveAnResult" ("Enum"), error in (no error)=w933) -> (error out=w931:errorcluster)  [unwired: 1 in, 2 out]
      }
      event "CalVar_Cal": Value Change {
        n548 = event-data() -> ()  [unwired: 1 in, 1 out]
        n549 = Enqueue Element(queue=w937, element=T12."Calvar3Open" ("Enum"), error in (no error)=w936) -> (error out=w934:errorcluster)  [unwired: 1 in, 2 out]
      }
      event "Calibration Data Location": Value Change {
        n550 = event-data() -> ()  [unwired: 1 in, 1 out]
        n551 = Enqueue Element(queue=w941, element=T12."CalDataOpen" ("Enum"), error in (no error)=w940) -> (error out=w938:errorcluster)  [unwired: 1 in, 2 out]
      }
      event "Calibration Data:": Double Click {
        n552 = event-data() -> ()  [unwired: 1 in, 1 out]
        n553 = Enqueue Element(queue=w945, element=T12."CalGrpOpen" ("Enum"), error in (no error)=w944) -> (error out=w943:errorcluster)  [unwired: 1 in, 2 out]
      }
      event "Axis": Value Change {
        n554 = event-data() -> ()  [unwired: 1 in, 1 out]
        n555 = Enqueue Element(queue=w949, element=T12."CalGrpOpen" ("Enum"), error in (no error)=w948) -> (error out=w947:errorcluster)  [unwired: 1 in, 2 out]
      }
      event "btn_addAvg": Value Change {
        n556 = event-data() -> ()  [unwired: 1 in, 1 out]
        n557 = Enqueue Element(queue=w952, element=T12."AddAvg" ("Enum"), error in (no error)=w951) -> (error out=w953:errorcluster)  [unwired: 1 in, 2 out]
      }
      event "테이블 컨트롤": Mouse Up {
        n558 = event-data() -> ("Coords.Horizontal"=→"Horizontal 2":i32, "Coords.Vertical"=→"Vertical 2":i32)  [unwired: 1 in]
      }
      event "btn_rmvAvg": Value Change {
        n559 = event-data() -> ()  [unwired: 1 in, 1 out]
        n560 = Enqueue Element(queue=w958, element=T12."RmvAvg" ("Enum"), error in (no error)=w957) -> (error out=w959:errorcluster)  [unwired: 1 in, 2 out]
      }
      event "btn_Calculate": Value Change {
        n561 = event-data() -> ()  [unwired: 1 in, 1 out]
        n562 = Enqueue Element(queue=w961, element=T12."CalCalvar" ("Enum"), error in (no error)=w962) -> (error out=w963:errorcluster)  [unwired: 1 in, 2 out]
      }
      event "btn_add2list": Value Change {
        n563 = event-data() -> ()  [unwired: 1 in, 1 out]
        n564 = Enqueue Element(queue=w966, element=T12."AddVar" ("Enum"), error in (no error)=w965) -> (error out=w967:errorcluster)  [unwired: 1 in, 2 out]
      }
      event "btn_save": Value Change {
        n565 = event-data() -> ()  [unwired: 1 in, 1 out]
        n566 = Enqueue Element(queue=w971, element=T12."SaveVar" ("Enum"), error in (no error)=w970) -> (error out=w969:errorcluster)  [unwired: 1 in, 2 out]
      }
      event "btn_up": Value Change {
        n567 = event-data() -> ()  [unwired: 1 in, 1 out]
        n568 = Enqueue Element(queue=w975, element=T12."Up" ("Enum"), error in (no error)=w974) -> (error out=w973:errorcluster)  [unwired: 1 in, 2 out]
      }
      event "btn_dn": Value Change {
        n569 = event-data() -> ()  [unwired: 1 in, 1 out]
        n570 = Enqueue Element(queue=w979, element=T12."Dn" ("Enum"), error in (no error)=w978) -> (error out=w977:errorcluster)  [unwired: 1 in, 2 out]
      }
      event "btn_del": Value Change {
        n571 = event-data() -> ()  [unwired: 1 in, 1 out]
        n572 = Enqueue Element(queue=w983, element=T12."Del" ("Enum"), error in (no error)=w982) -> (error out=w981:errorcluster)  [unwired: 1 in, 2 out]
      }
      event "Close": Value Change {
        n573 = event-data() -> ()  [unwired: 1 in, 1 out]
      }
      event "Grp_ExtVel_Hor": Cursor Release {
        n574 = event-data() -> ()  [unwired: 1 in, 5 out]
        n575 = property on="Grp_ExtVel_Hor" class="WFGraph (strict)"() -> ("CrsrList"=w993:T20)  [unwired: 2 in, 2 out]
        n576 = Index Array(array=w993) -> (element #1=w992:T21, element #2=w991:T21)  [unwired: 2 in]
        n577 = Unbundle By Name(w992) -> ("Position.X"=w989:dbl)
        n578 = Unbundle By Name(w991) -> ("Position.X"=w990:dbl)
        n579 = Subtract(x=w989, y=w990) -> (x-y=w988:dbl)
        n580 = local write "Decaytime (Sec)"(w988) -> ()
      }
    }
    n581 = Unbundle By Name(w833) -> ("status"=w828:bool)
    n582 = Unbundle By Name(w827) -> ("status"=w826:bool)
    n583 = Unbundle By Name(w825) -> ("status"=w824:bool)
    n584 = Compound Arithmetic op=OR(w828, w826, w824, w835) -> (w834:bool)
  }
  n585 = while {
    tunnel: w21 -> [w1000]
    tunnel: w7 -> [w996]
    shift-right: [w994] -> _
    shift-left: enum16{"Idle", "Tracking"}."Idle" ("Enum") -> [w995]
    stop <- w997 stop-if-true
    # "Video Analysis"
    n586 = Dequeue Element(queue=w1000) -> (element=w998:T13, error out=w999:errorcluster)  [unwired: 2 in, 2 out]
    n587 = case shown="No Error" w999 {
      tunnel: w998 -> [w1004 _]
      tunnel: [_ TRUE] -> w997
      tunnel: w996 -> [w1003 _]
      tunnel: w995 -> [w1002 w1309]
      tunnel: [w1001 w1309] -> w994
      frame No Error {
        n588 = case shown="\"Tracking\"" w1002 {
          tunnel: w1004 -> [w1007 _]
          tunnel: w1003 -> [w1005 w1140]
          tunnel: [w1006 enum16{"Idle", "Tracking"}."Idle" ("Enum")] -> w1001
          frame "Idle", Default {
            n589 = case shown="\"CalDateChange\"" w1007 {
              tunnel: [enum16{"Idle", "Tracking"}."Idle" ("Enum") enum16{"Idle", "Tracking"}."Idle" ("Enum") enum16{"Idle", "Tracking"}."Idle" ("Enum") enum16{"Idle", "Tracking"}."Idle" ("Enum") enum16{"Idle", "Tracking"}."Tracking" ("Enum") enum16{"Idle", "Tracking"}."Idle" ("Enum")] -> w1006
              tunnel: w1005 -> [w1008 _ _ w1071 _ _]
              frame "VideoFileOpen", Default {
                n590 = Unbundle(w1008) -> ("New Image"=w1011:T9, "New Image"=w1010:T9)  [unwired: 3 out]
                n591 = stacked-sequence {
                  tunnel: w1011 -> [_ _ w1033]
                  tunnel: w1010 -> [_ _ w1015]
                  frame #0 {
                    w1013 = 0.0 ("Data Entry Limits:Maximum")
                    n592 = property on="FrameNum" class="Slide (strict)"("Scale.Minimum"=w1013, "Minimum"=w1013) -> ()  [unwired: 2 in, 2 out]
                    n593 = property on="btn_Detect" class="Bool"("DisabledEnum"=T19."Enabled" ("Disabled")) -> ()  [unwired: 2 in, 2 out]
                  }
                  frame #1 {
                    n594 = invoke on="FrameNum" class="Slide (strict)" method="Reinit To Default"() -> ()  [unwired: 3 in, 3 out]
                    n595 = invoke on="Freq:" class="Str" method="Reinit To Default"() -> ()  [unwired: 3 in, 3 out]
                    n596 = invoke on="comp_XY" class="WFChart (strict)" method="Reinit To Default"() -> ()  [unwired: 3 in, 3 out]
                    n597 = invoke on="Detection Sensitivity" class="Slide (strict)" method="Reinit To Default"() -> ()  [unwired: 3 in, 3 out]
                    n598 = invoke on="Img_Org" class="ImageControl" method="Reinit To Default"() -> ()  [unwired: 3 in, 3 out]
                    n599 = invoke on="FPS:" class="DigNum (strict)" method="Reinit To Default"() -> ()  [unwired: 3 in, 3 out]
                    n600 = property on="comp_XY" class="WFChart (strict)"("History Data"=cluster{"mean":dbl, "mean":dbl, "Angle":sgl}[] []) -> ()  [unwired: 2 in, 2 out]
                  }
                  frame #2 {
                    n601 = local read "Video File"() -> (w1019:path)
                    n602 = local read "BCGTD"() -> (w1024:T8)
                    n603 = call "IMAQ AVI Open"("AVI Path"=w1019) -> ("error out"=w1030:errorcluster, "Avi Refnum"=w1035:T27)  [unwired: 9 in]
                    n604 = property on="FrameNum" class="Slide (strict)"() -> ("Value"=w1026:u32)  [unwired: 2 in, 2 out]
                    n605 = Unbundle(w1024) -> ("Brightness"=w1023:sgl, "Contrast"=w1022:sgl, "Gamma"=w1021:sgl)  [unwired: 1 out]
                    n606 = call "IMAQ AVI Get Info"("error in (no error)"=w1030, "Avi Refnum"=w1035) -> ("error out"=w1029:errorcluster, "Number of Frames"=w1028:u32, "Avi Refnum (duplicate)"=w1034:T27, "Frame Data"=w1018:T28)  [unwired: 6 out]
                    n607 = Unbundle By Name(w1018) -> ("framesPerSecond"=w1017:u32)
                    n608 = Bundle("Brightness"=w1023, "Contrast"=w1022, "Gamma"=w1021) -> (w1020:T29)  [unwired: 1 in]
                    n609 = local write "FPS:"(w1017) -> ()
                    n610 = Decrement(x=w1028) -> (x-1=w1027:u32)
                    n611 = call "IMAQ AVI Read Frame"("error in (no error)"=w1029, "Frame Number"=w1026, "Image"=w1033, "Avi Refnum"=w1034) -> ("error out"=w1031:errorcluster, "Image Out"=w1025:T9, "Avi Refnum (duplicate)"=w1032:T27)  [unwired: 4 in, 1 out]
                    n612 = call "IMAQ BCGLookup"("Image Src"=w1025, "BCG Values"=w1020, "Image Dst"=w1015) -> ("Image Dst Out"=w1016:T9)  [unwired: 4 in, 1 out]
                    n613 = call "IMAQ AVI Close"("error in (no error)"=w1031, "Avi Refnum"=w1032) -> ()  [unwired: 9 in, 1 out]
                    n614 = property on="FrameNum" class="Slide (strict)"("Maximum"=w1027, "Scale.Maximum"=w1027) -> ()  [unwired: 2 in, 2 out]
                    n615 = local write "Img_Org"(w1016) -> ()
                  }
                }
              }
              frame "CalvarOpen" {
                n616 = local read "CalVar_VA"() -> (w1037:path)
                n617 = call-poly <vilib>:"Read From Spreadsheet File.vi"("delimiter (\\t)"="," ("delimiter (\\t)"), "file path (dialog if empty)"=w1037) -> ("all rows"=w1045:string[][])  [unwired: 5 in, 4 out]
                n618 = Index Array(array=w1045, index (col) #1=0 ("disabled index (col)")) -> (element #1=w1043:string[], element #2=w1048:string[], element #3=w1052:string[])  [unwired: 5 in]
                n619 = Reverse 1D Array(array=w1043) -> (reversed array=w1047:string[])
                n620 = Reverse 1D Array(array=w1048) -> (reversed array=w1049:string[])
                n621 = Reverse 1D Array(array=w1052) -> (reversed array=w1054:string[])
                n622 = Index Array(array=w1054, index=0) -> (element=w1055:string)
                n623 = Index Array(array=w1047, index=0) -> (element=w1040:string)
                n624 = Index Array(array=w1049, index=0) -> (element=w1051:string)
                n625 = property on="Cal_Val:" class="Ring (strict)"("Strings []"=w1047) -> (error out=w1042:errorcluster)  [unwired: 2 in, 1 out]
                n626 = property on="Cal_Val:" class="Ring (strict)"(error in=w1042, "RingText.Text"=w1040) -> ()  [unwired: 1 in, 2 out]
                n627 = Fract/Exp String To Number(string=w1051) -> (number=w1039:dbl)  [unwired: 3 in, 1 out]
                n628 = Fract/Exp String To Number(string=w1055) -> (number=w1038:dbl)  [unwired: 3 in, 1 out]
                n629 = local write "Y-axis"(w1038) -> ()
                n630 = local write "X-axis"(w1039) -> ()
              }
              frame "CalDateChange" {
                n631 = local read "CalVar_VA"() -> (w1057:path)
                n632 = local read "Cal_Val:"() -> (w1058:u16)
                n633 = call-poly <vilib>:"Read From Spreadsheet File.vi"("delimiter (\\t)"="," ("delimiter (\\t)"), "file path (dialog if empty)"=w1057) -> ("all rows"=w1060:dbl[][])  [unwired: 5 in, 4 out]
                n634 = Index Array(array=w1060, index (col) #1=1 ("disabled index (col)")) -> (element #1=w1064:dbl[], element #2=w1066:dbl[])  [unwired: 3 in]
                n635 = Reverse 1D Array(array=w1064) -> (reversed array=w1065:dbl[])
                n636 = Reverse 1D Array(array=w1066) -> (reversed array=w1067:dbl[])
                n637 = Index Array(array=w1065, index=w1058) -> (element=w1062:dbl)
                n638 = Index Array(array=w1067, index=w1058) -> (element=w1063:dbl)
                n639 = local write "X-axis"(w1062) -> ()
                n640 = local write "Y-axis"(w1063) -> ()
              }
              frame "Adj_BCGTD" {
                n641 = Unbundle(w1071) -> ("New Image"=w1072:T9, "New Image"=w1069:T9)  [unwired: 3 out]
                n642 = local read "BCGTD"() -> (w1077:T8)
                n643 = Unbundle(w1077) -> ("Brightness"=w1076:sgl, "Contrast"=w1075:sgl, "Gamma"=w1074:sgl)  [unwired: 1 out]
                n644 = local read "Video File"() -> (w1068:path)
                n645 = Bundle("Brightness"=w1076, "Contrast"=w1075, "Gamma"=w1074) -> (w1073:T29)  [unwired: 1 in]
                n646 = Not Equal?(x=w1068, y=path "") -> (x != y?=w1078:bool)
                n647 = case shown="True" w1078 {
                  tunnel: w1073 -> [_ w1085]
                  tunnel: w1072 -> [_ w1082]
                  tunnel: w1069 -> [_ w1081]
                  frame False {
                  }
                  frame True {
                    n648 = property on="Image Flip" class="Ring (strict)"() -> ("Value"=w1080:u32)  [unwired: 2 in, 2 out]
                    n649 = case shown="3, Default" w1080 {
                      tunnel: w1082 -> [w1087 w1093 w1096 w1098]
                      tunnel: [w1086 w1092 w1094 w1098] -> w1083
                      tunnel: w1080 -> [w1089 w1091 w1095 _]
                      tunnel: w1081 -> [w1088 w1090 w1097 _]
                      frame 0 {
                        n650 = call "IMAQ Symmetry"("Type of Symmetry"=w1089, "Image Dst"=w1088, "Image Src"=w1087) -> ("Image Dst Out"=w1086:T9)  [unwired: 2 in, 1 out]
                      }
                      frame 1 {
                        n651 = call "IMAQ Symmetry"("Type of Symmetry"=w1091, "Image Dst"=w1090, "Image Src"=w1093) -> ("Image Dst Out"=w1092:T9)  [unwired: 2 in, 1 out]
                      }
                      frame 2 {
                        n652 = call "IMAQ Symmetry"("Type of Symmetry"=w1095, "Image Dst"=w1097, "Image Src"=w1096) -> ("Image Dst Out"=w1094:T9)  [unwired: 2 in, 1 out]
                      }
                      frame 3, Default {
                      }
                    }
                    n653 = call "Vision Assistant4"("Image In"=w1083, "Image Dst"=w1081, "BCG Values (Brightness 1)"=w1085) -> ("Image Out"=w1084:T9)  [unwired: 23 in, 1 out]
                    n654 = local write "Img_Org"(w1084) -> ()
                  }
                }
              }
              frame "StartTrack" {
              }
              frame "SaveResult" {
                n655 = Two Button Dialog(message="Are you sure to save analyzed result in a file?", 1:"No" ("F button name (\"Cancel\")"), 2:"Yes" ("T button name (\"OK\")")) -> (T button?=w1101:bool)
                n656 = case shown="True" w1101 {
                  frame False {
                  }
                  frame True {
                    n657 = stacked-sequence {
                      seq-local: [w1117 _] -> [_ w1134]
                      frame #0 {
                        n658 = property on="Video File" class="Path"() -> ("Text.Text"=w1121:string)  [unwired: 2 in, 2 out]
                        n659 = Search and Replace String(input string=w1121, search string=".avi" ("검색 문자열"), replace string="_VT.csv" ("대체 문자열(\"\")")) -> (result string=w1124:string)  [unwired: 5 in, 3 out]
                        n660 = String To Path(string=w1124) -> (path=w1117:path)
                        n661 = call-poly <vilib>:"Read From Spreadsheet File.vi"("delimiter (\\t)"="," ("delimiter (\\t)"), "transpose (no:F)"=TRUE, "file path (dialog if empty)"=w1117) -> ("all rows"=w1107:dbl[][])  [unwired: 4 in, 4 out]
                        n662 = property on="comp_XY" class="WFChart (strict)"() -> ("History Data"=w1126:cluster{"mean":dbl, "mean":dbl, "Angle":sgl}[])  [unwired: 2 in, 2 out]
                        n663 = Index Array(array=w1107) -> (element #1=w1106:dbl[], element #2=w1105:dbl[])  [unwired: 4 in]
                        n664 = for {
                          tunnel: w1126 -> [w1132] mode=indexing
                          tunnel: [w1130] -> w1116 mode=indexing
                          tunnel: [w1129] -> w1112 mode=indexing
                          tunnel: [w1131] -> w1109 mode=indexing
                          workers-P: _ -> [_]
                          n665 = Unbundle(w1132) -> ("mean"=w1130:dbl, "mean"=w1129:dbl, "Angle"=w1131:sgl)
                        }
                        n666 = Index Array(array=w1116) -> (element=w1115:dbl)  [unwired: 1 in]
                        n667 = Index Array(array=w1112) -> (element=w1113:dbl)  [unwired: 1 in]
                        n668 = Index Array(array=w1109) -> (element=w1110:sgl)  [unwired: 1 in]
                        n669 = Subtract(x=w1116, y=w1115) -> (x-y=w1114:dbl[])
                        n670 = Subtract(x=w1112, y=w1113) -> (x-y=w1111:dbl[])
                        n671 = Subtract(x=w1109, y=w1110) -> (x-y=w1108:sgl[])
                        n672 = Build Array(w1106, w1105, w1114, w1111, w1108) -> (w1125:dbl[][])
                        n673 = call "다이나믹 데이터로 변환"("2D Array"=w1125) -> ("Dynamic Data Type"=w1119:dynamicdata)  [unwired: 3 in]
                        n674 = call "Build Table"("Signals"=w1119) -> ("Table"=w1127:string[][])  [unwired: 4 in, 6 out]
                        n675 = call-poly <vilib>:"Write To Spreadsheet File.vi"("delimiter (\\t)"="," ("delimiter (\\t)"), "2D data"=w1127, "file path (dialog if empty)"=w1117) -> ()  [unwired: 5 in, 1 out]
                      }
                      frame #1 {
                        n676 = Path To String(path=w1134) -> (string=w1135:string)
                        n677 = Concatenate Strings("Video analysis has been saved as " ("message"), w1135) -> (w1133:string)
                        n678 = One Button Dialog(message=w1133) -> ()  [unwired: 1 in, 1 out]
                      }
                    }
                  }
                }
              }
            }
          }
          frame "Tracking" {
            n679 = Unbundle(w1140) -> ("New Image"=w1144:T9, "New Image"=w1143:T9, "New Image"=w1142:T9, "New Image"=w1137:T9, "New Image"=w1141:T9)
            n680 = property on="Video File" class="Path"() -> (error out=w1152:errorcluster, "Value"=w1151:path)  [unwired: 2 in, 1 out]
            n681 = property on="btn_Start" class="Bool"("BoolText.Text"="Analyzing..." ("캡션.텍스트"), "DisabledEnum"=T19."Disabled and Grayed Out" ("비활성화")) -> ()  [unwired: 2 in, 2 out]
            n682 = property on="btn_Pause" class="Bool (strict)"("DisabledEnum"=T19."Enabled" ("비활성화")) -> ()  [unwired: 2 in, 2 out]
            n683 = call "IMAQ AVI Open"("error in (no error)"=w1152, "AVI Path"=w1151) -> ("error out"=w1148:errorcluster, "Avi Refnum"=w1147:T27)  [unwired: 8 in]
            n684 = while {
              tunnel: w1148 -> [w1168]
              tunnel: w1144 -> [w1167]
              tunnel: w1147 -> [w1166]
              tunnel: [w1165] -> w1146
              tunnel: w1143 -> [w1164]
              tunnel: w1142 -> [w1163]
              tunnel: w1141 -> [w1162]
              tunnel: [w1156] -> w1138
              tunnel: w1137 -> [w1154]
              i -> [w1160]
              stop <- w1157 stop-if-true
              n685 = property on="FrameNum" class="Slide (strict)"() -> ("Maximum"=w1161:dbl)  [unwired: 2 in, 2 out]
              n686 = case shown="False" "btn_Pause" {
                tunnel: w1168 -> [w1179 w1301]
                tunnel: w1167 -> [w1178 _]
                tunnel: w1166 -> [w1177 w1302]
                tunnel: [w1176 w1302] -> w1165
                tunnel: w1164 -> [w1175 _]
                tunnel: w1163 -> [w1174 _]
                tunnel: w1162 -> [w1173 _]
                tunnel: w1160 -> [w1172 _]
                tunnel: [w1171 w1301] -> w1156
                tunnel: [w1170 w1301] -> w1155
                tunnel: w1154 -> [w1169 _]
                frame False {
                  n687 = stacked-sequence {
                    seq-local: [_ w1214 _] -> [_ _ w1253]
                    seq-local: [_ w1211 _] -> [_ _ w1239]
                    tunnel: w1179 -> [w1195 _ _]
                    tunnel: [w1194 _ _] -> w1176
                    tunnel: w1172 -> [w1190 _ _]
                    tunnel: w1178 -> [w1193 _ _]
                    tunnel: w1177 -> [w1192 _ _]
                    tunnel: w1175 -> [w1182 w1213 w1252]
                    tunnel: w1174 -> [_ w1228 _]
                    tunnel: w1173 -> [_ _ _]
                    tunnel: [w1191 _ _] -> w1171
                    tunnel: [w1191 _ _] -> w1170
                    tunnel: w1169 -> [_ _ w1250]
                    frame #0 {
                      # "Image Aquisition"
                      n688 = local read "BCGTD"() -> (w1189:T8)
                      n689 = Unbundle(w1189) -> ("Brightness"=w1188:sgl, "Contrast"=w1187:sgl, "Gamma"=w1186:sgl)  [unwired: 1 out]
                      n690 = Bundle("Brightness"=w1188, "Contrast"=w1187, "Gamma"=w1186) -> (w1184:T29)  [unwired: 1 in]
                      n691 = call "IMAQ AVI Read Frame"("error in (no error)"=w1195, "Frame Number"=w1190, "Image"=w1193, "Avi Refnum"=w1192) -> ("error out"=w1191:errorcluster, "Image Out"=w1183:T9, "Avi Refnum (duplicate)"=w1194:T27)  [unwired: 4 in, 1 out]
                      n692 = case shown="1" "Image Flip" {
                        tunnel: w1183 -> [w1197 w1203 w1206 w1208]
                        tunnel: [w1196 w1202 w1204 w1208] -> w1181
                        tunnel: "Image Flip" -> [w1199 w1201 w1205 _]
                        tunnel: w1182 -> [w1198 w1200 w1207 _]
                        frame 0 {
                          n693 = call "IMAQ Symmetry"("Type of Symmetry"=w1199, "Image Dst"=w1198, "Image Src"=w1197) -> ("Image Dst Out"=w1196:T9)  [unwired: 2 in, 1 out]
                        }
                        frame 1 {
                          n694 = call "IMAQ Symmetry"("Type of Symmetry"=w1201, "Image Dst"=w1200, "Image Src"=w1203) -> ("Image Dst Out"=w1202:T9)  [unwired: 2 in, 1 out]
                        }
                        frame 2 {
                          n695 = call "IMAQ Symmetry"("Type of Symmetry"=w1205, "Image Dst"=w1207, "Image Src"=w1206) -> ("Image Dst Out"=w1204:T9)  [unwired: 2 in, 1 out]
                        }
                        frame 3, Default {
                        }
                      }
                      n696 = call "Vision Assistant"("Image In"=w1181, "Image Dst"=w1182, "BCG Values (Brightness 1)"=w1184) -> ("Image Out"=w1185:T9)  [unwired: 23 in, 1 out]
                      n697 = local write "FrameNum"(w1190) -> ()
                      n698 = local write "Img_Org"(w1185) -> ()
                    }
                    frame #1 {
                      w1227 = u16 0 items=["Shift Invariant", "Rotation Invariant"] ("Match Mode (Pattern Matching 1)")
                      # "Image Processing"
                      n699 = local read "BCGTD"() -> (w1230:T8)
                      n700 = Unbundle(w1230) -> ("Detection Sensitivity"=w1212:sgl)  [unwired: 3 out]
                      n701 = call "PatternMatching.vi"("Image In"=w1213, "Match Mode (Pattern Matching 1)"=w1227, "Number of Matches Requested (Pattern Matching 1)"=1, "Minimum Match Score (Pattern Matching 1)"=w1212, "Marker Image"=w1228) -> ("Matches (Pattern Matching 1)"=w1216:T30, "Number of Matches (Pattern Matching 1)"=w1209:i32)  [unwired: 18 in, 3 out]
                      n702 = Not Equal To 0?(x=w1209) -> (x != 0?=w1210:bool)
                      n703 = Index Array(array=w1216) -> (element=w1211:T31)  [unwired: 1 in]
                      n704 = case shown="False" w1210 {
                        frame False {
                          n705 = property on="Marker Detection" class="Bool (strict)"("Value"=FALSE ("Number of Matches (Pattern Matching 1)")) -> ()  [unwired: 2 in, 2 out]
                        }
                        frame True {
                          "Number of Matches (Pattern Matching 1)" <- TRUE ("Number of Matches (Pattern Matching 1)")
                        }
                      }
                      n706 = Unbundle(w1211) -> ("Bounding Box"=w1226:cluster{"x":sgl, "y":sgl}[])  [unwired: 4 out]
                      n707 = Index Array(array=w1226) -> (element #1=w1225:cluster{"x":sgl, "y":sgl}, element #2=w1224:cluster{"x":sgl, "y":sgl}, element #3=w1223:cluster{"x":sgl, "y":sgl}, element #4=w1222:cluster{"x":sgl, "y":sgl})  [unwired: 5 in, 1 out]
                      n708 = Unbundle(w1225) -> ("x"=w1221:sgl, "y"=w1220:sgl)
                      n709 = Unbundle(w1224) -> ("x"=w1219:sgl)  [unwired: 1 out]
                      n710 = Unbundle(w1223) -> ("y"=w1218:sgl)  [unwired: 1 out]
                      n711 = Unbundle(w1222) -> ()  [unwired: 2 out]
                      n712 = Bundle By Name(cluster=T26 {"Left"=0, "Top"=0, "Right"=0, "Bottom"=0, "Rotation"=0.0} ("Rectangle"), "Left"=w1221, "Top"=w1220, "Right"=w1219, "Bottom"=w1218, "Rotation"=sgl 0.0 ("원소")) -> (w1214:T26)
                      n713 = local write "Img_Org"(w1213) -> ()
                    }
                    frame #2 {
                      w1249 = 15.0 ("y")
                      n714 = case shown="False" "Round Marker?" {
                        tunnel: w1253 -> [w1295 _]
                        tunnel: w1252 -> [w1293 w1299]
                        tunnel: w1250 -> [w1277 _]
                        tunnel: [w1273 w1299] -> w1242
                        tunnel: [w1254 w1296] -> w1233
                        tunnel: [w1269 _] -> w1238
                        tunnel: [w1255 w1297] -> w1234
                        tunnel: w1239 -> [w1256 w1300]
                        frame False {
                          n715 = call "IMAQ Convert Rectangle to ROI"("Rectangle"=w1295) -> ("ROI Descriptor"=w1294:T32)  [unwired: 8 in, 1 out]
                          n716 = call "Vision Assistant3"("Image In"=w1293, "Image Dst"=w1277, "ROI Descriptor (Find Straight Edge 1)"=w1294, "Options (Find Straight Edge 1)"="Marker Edge 1", "Fit Options (Find Straight Edge 1)"="Fit Options (Find Straight Edge 1)", "ROI Descriptor (Copy of Find Straight Edge 1)"=w1294, "Options (Copy of Find Straight Edge 1)"="Marker Edge 2", "Fit Options (Copy of Find Straight Edge 1)"="Fit Options (Find Straight Edge 2)", "ROI Descriptor (Copy of Copy of Find Straight Edge 1)"=w1294, "Options (Copy of Copy of Find Straight Edge 1)"="Marker Edge 3", "Fit Options (Copy of Copy of Find Straight Edge 1)"="Fit Options (Find Straight Edge 3)") -> ("Image Out"=w1273:T9, "Straight Edge (Find Straight Edge 1)"=w1292:T33, "Straight Edge (Copy of Find Straight Edge 1)"=w1291:T33, "Straight Edge (Copy of Copy of Find Straight Edge 1)"=w1290:T33)  [unwired: 12 in, 1 out]
                          n717 = Unbundle By Name(w1292) -> ("Angle (Pixel)"=w1260:dbl, "Point1 (Pixels).X"=w1289:sgl, "Point2 (Pixels).X"=w1288:sgl, "Point1 (Pixels).Y"=w1283:sgl, "Point2 (Pixels).Y"=w1282:sgl)
                          n718 = Unbundle By Name(w1291) -> ("Angle (Pixel)"=w1259:dbl, "Point1 (Pixels).X"=w1287:sgl, "Point2 (Pixels).X"=w1286:sgl, "Point1 (Pixels).Y"=w1281:sgl, "Point2 (Pixels).Y"=w1280:sgl)
                          n719 = Unbundle By Name(w1290) -> ("Angle (Pixel)"=w1258:dbl, "Point1 (Pixels).X"=w1285:sgl, "Point2 (Pixels).X"=w1284:sgl, "Point1 (Pixels).Y"=w1279:sgl, "Point2 (Pixels).Y"=w1278:sgl)
                          n720 = Build Array(w1289, w1288, w1287, w1286, w1285, w1284) -> (w1267:sgl[])
                          n721 = Build Array(w1283, w1282, w1281, w1280, w1279, w1278) -> (w1265:sgl[])
                          n722 = Build Array(w1260, w1259, w1258) -> (w1263:dbl[])
                          n723 = Search 1D Array(1D array=w1267, element=sgl 0.0) -> (index of element=w1262:i32)  [unwired: 1 in]
                          n724 = Unbundle(w1256) -> ("Position"=w1257:cluster{"x":sgl, "y":sgl})  [unwired: 4 out]
                          n725 = Delete From Array(array=w1267, index=w1262) -> (array with subset deleted=w1266:sgl[])  [unwired: 1 in, 1 out]
                          n726 = Delete From Array(array=w1265, index=w1262) -> (array with subset deleted=w1264:sgl[])  [unwired: 1 in, 1 out]
                          n727 = Delete From Array(array=w1263, index=w1262) -> (array with subset deleted=w1261:dbl[])  [unwired: 1 in, 1 out]
                          n728 = Unbundle(w1257) -> ("x"=w1255:sgl, "y"=w1254:sgl)
                          n729 = call-poly <vilib>:"Mean.vi"("X"=w1264) -> ()  [unwired: 2 out]
                          n730 = call-poly <vilib>:"Mean.vi"("X"=w1266) -> ()  [unwired: 2 out]
                          n731 = call-poly <vilib>:"Mean.vi"("X"=w1261) -> ("mean"=w1269:dbl)  [unwired: 1 out]
                        }
                        frame True {
                          n732 = Unbundle(w1300) -> ("Position"=w1298:cluster{"x":sgl, "y":sgl})  [unwired: 4 out]
                          n733 = Unbundle(w1298) -> ("x"=w1297:sgl, "y"=w1296:sgl)
                        }
                      }
                      n734 = Add(x=w1234, y=w1249) -> (x+y=w1246:dbl)
                      n735 = Add(x=w1233, y=w1249) -> (x+y=w1245:dbl)
                      n736 = Subtract(x=w1234, y=w1249) -> (x-y=w1248:dbl)
                      n737 = Subtract(x=w1233, y=w1249) -> (x-y=w1247:dbl)
                      n738 = Negate(x=w1234) -> (-x=w1237:sgl)
                      n739 = Negate(x=w1233) -> (-x=w1236:sgl)
                      n740 = Negate(x=w1238) -> (-x=w1235:dbl)
                      n741 = Bundle(w1248, w1247, w1246, w1245) -> (w1244:cluster{dbl, dbl, dbl, dbl})  [unwired: 1 in]
                      n742 = call "IMAQ Overlay Oval"("Color"=u32 6618880, "Bounding Rectangle"=w1244, "Image"=w1242) -> ("Image Out"=w1243:T9)  [unwired: 7 in, 1 out]
                      n743 = local write "Img_Mod"(w1243) -> ()
                      n744 = Bundle(w1237, w1236, w1235) -> (w1251:cluster{sgl, sgl, dbl})  [unwired: 1 in]
                      n745 = local write "comp_XY"(w1251) -> ()
                    }
                  }
                }
                frame True {
                  n746 = while {
                    stop <- w1303 continue-if-true
                    n747 = local read "btn_Pause"() -> (w1303:bool)
                    n748 = Wait (ms)(milliseconds to wait=u32 10) -> ()  [unwired: 1 out]
                  }
                }
              }
              n749 = Less Or Equal?(x=w1161, y=w1160) -> (x <= y?=w1159:bool)
              n750 = Compound Arithmetic op=OR(w1155, "btn_Stop", w1159) -> (w1157:bool)
              n751 = case shown="True" w1157 {
                frame False {
                }
                frame True {
                  n752 = stacked-sequence {
                    frame #0 {
                      n753 = property on="FrameNum" class="Slide (strict)"("DisabledEnum"=T19."Enabled" ("비활성화")) -> ()  [unwired: 2 in, 2 out]
                    }
                    frame #1 {
                      n754 = property on="btn_Start" class="Bool"("BoolText.Text"="Start" ("캡션.텍스트"), "DisabledEnum"=T19."Enabled" ("비활성화")) -> ()  [unwired: 2 in, 2 out]
                    }
                    frame #2 {
                      w1308 = T19."Enabled" ("Disabled")
                      n755 = property on="btn_SaveResult" class="Bool"("DisabledEnum"=w1308) -> ()  [unwired: 2 in, 2 out]
                      n756 = property on="btn_Reset" class="Bool"("DisabledEnum"=w1308) -> ()  [unwired: 2 in, 2 out]
                    }
                  }
                }
              }
            }
            n757 = call "IMAQ AVI Close"("error in (no error)"=w1138, "Avi Refnum"=w1146) -> ()  [unwired: 9 in, 1 out]
          }
        }
      }
      frame Error {
      }
    }
  }
  n758 = Release Queue(queue=w21, error in (no error)=w20) -> ()  [unwired: 1 in, 3 out]
  n759 = Release Queue(queue=w3, error in (no error)=w15) -> ()  [unwired: 1 in, 3 out]
  n760 = Release Queue(queue=w4, error in (no error)=w14) -> ()  [unwired: 1 in, 3 out]
  n761 = stacked-sequence {
    frame #0 {
      n762 = control-ref of="This VI"() -> (w1311:refnum<vi>)
      n763 = invoke class="VI" method="Default Vals.Reinit All"(reference=w1311) -> ()  [unwired: 2 in, 3 out]
    }
    frame #1 {
      n764 = property on="Video File" class="Path"() -> ("Value"=w1313:path)  [unwired: 2 in, 2 out]
      n765 = Not Equal?(x=w1313, y=path "") -> (x != y?=w1312:bool)
      n766 = case shown="False" w1312 {
        frame False {
          w1315 = 0.0 ("Data Entry Limits:Maximum")
          w1316 = T19."Disabled and Grayed Out" ("Disabled")
          n767 = property on="btn_Detect" class="Bool"("DisabledEnum"=w1316) -> ()  [unwired: 2 in, 2 out]
          n768 = property on="btn_Pause" class="Bool (strict)"("DisabledEnum"=w1316) -> ()  [unwired: 2 in, 2 out]
          n769 = property on="btn_Reset" class="Bool"("DisabledEnum"=w1316) -> ()  [unwired: 2 in, 2 out]
          n770 = property on="btn_SaveResult" class="Bool"("DisabledEnum"=w1316) -> ()  [unwired: 2 in, 2 out]
          n771 = property on="btn_Start" class="Bool"("DisabledEnum"=w1316) -> ()  [unwired: 2 in, 2 out]
          n772 = property on="FrameNum" class="Slide (strict)"("DisabledEnum"=w1316, "Scale.Minimum"=w1315, "Minimum"=w1315) -> ()  [unwired: 2 in, 2 out]
        }
        frame True {
          w1318 = 0.0 ("Data Entry Limits:Maximum")
          w1317 = T19."Enabled" ("Disabled")
          n773 = property on="FrameNum" class="Slide (strict)"("DisabledEnum"=w1317, "Scale.Minimum"=w1318, "Minimum"=w1318) -> ()  [unwired: 2 in, 2 out]
          n774 = property on="btn_Detect" class="Bool"("DisabledEnum"=w1317) -> ()  [unwired: 2 in, 2 out]
        }
      }
    }
    frame #2 {
      n775 = call <vilib>:"Application Directory.vi"() -> ("Application Directory"=w1337:path)
      n776 = Build Path(base path=w1337, name or relative path="calvar.csv") -> (appended path=w1319:path)
      n777 = call-poly <vilib>:"Read From Spreadsheet File.vi"("delimiter (\\t)"="," ("delimiter (\\t)"), "file path (dialog if empty)"=w1319) -> ("all rows"=w1339:string[][])  [unwired: 5 in, 4 out]
      n778 = local write "CalVar_Cal"(w1319) -> ()
      n779 = local write "CalVar_VA"(w1319) -> ()
      n780 = local write "CalVar_GA"(w1319) -> ()
      n781 = call-poly <vilib>:"Read From Spreadsheet File.vi"("delimiter (\\t)"="," ("delimiter (\\t)"), "file path (dialog if empty)"=w1319) -> ("all rows"=w1321:string[][])  [unwired: 5 in, 4 out]
      n782 = Index Array(array=w1339, index (col) #1=0 ("disabled index (col)")) -> (element #1=w1341:string[], element #2=w1335:string[], element #3=w1331:string[])  [unwired: 5 in]
      n783 = property on="CalList" class="MCListbox (strict)"("ItemNames"=w1321, "Value"=0 ("CalList")) -> ()  [unwired: 2 in, 2 out]
      n784 = Reverse 1D Array(array=w1341) -> (reversed array=w1324:string[])
      n785 = Reverse 1D Array(array=w1335) -> (reversed array=w1334:string[])
      n786 = Reverse 1D Array(array=w1331) -> (reversed array=w1329:string[])
      n787 = Index Array(array=w1329, index=0) -> (element=w1328:string)
      n788 = Index Array(array=w1324, index=0) -> (element=w1323:string)
      n789 = Index Array(array=w1334, index=0) -> (element=w1332:string)
      n790 = property on="Cal_Val: 2" class="Ring (strict)"("Strings []"=w1324) -> (error out=w1325:errorcluster)  [unwired: 2 in, 1 out]
      n791 = property on="Cal_Val:" class="Ring (strict)"("Strings []"=w1324) -> (error out=w1342:errorcluster)  [unwired: 2 in, 1 out]
      n792 = property on="Cal_Val:" class="Ring (strict)"(error in=w1342, "RingText.Text"=w1323) -> ()  [unwired: 1 in, 2 out]
      n793 = property on="Cal_Val: 2" class="Ring (strict)"(error in=w1325, "RingText.Text"=w1323) -> ()  [unwired: 1 in, 2 out]
      n794 = Fract/Exp String To Number(string=w1332) -> (number=w1326:dbl)  [unwired: 3 in, 1 out]
      n795 = Fract/Exp String To Number(string=w1328) -> (number=w1327:dbl)  [unwired: 3 in, 1 out]
      n796 = local write "Y-axis 2"(w1327) -> ()
      n797 = local write "X-axis 2"(w1326) -> ()
      n798 = local write "X-axis"(w1326) -> ()
      n799 = local write "Y-axis"(w1327) -> ()
    }
    frame #3 {
      w1346 = u32 16448250
      n800 = property on="comp_XY" class="WFChart (strict)"("BG Color"=w1346) -> (error out=w1345:errorcluster)  [unwired: 2 in, 1 out]
      n801 = property on="grph_Calibration" class="WFGraph (strict)"("BG Color"=w1346) -> ()  [unwired: 2 in, 2 out]
      n802 = property on="comp_XY" class="WFChart (strict)"(error in=w1345, "History Data"=cluster{"mean":dbl, "mean":dbl, "Angle":sgl}[] []) -> ()  [unwired: 1 in, 2 out]
    }
  }
  "comp_XY" <- cluster{"mean":dbl, "mean":dbl, "Angle":sgl} {"mean"=0.0, "mean"=0.0, "Angle"=0.0} ("output cluster")
